vi "EnFlo_Tunnel_Display.vi"(4 "End Time":dbl, 5 "Start Time":dbl, 6 "Channel Values":dbl[](array[numeric]) format="%.3f", 7 "Ch names":string[](array[string])) -> ()   [LabVIEW 2021]
uses:
  Anemometry Sub Vis/Data_plotting_vis/File_Template_Clus.ctl
  Data plotting/subVIs/Dispose_Channel.ctl
  Anemometry Sub Vis/Controls/Global_mode.ctl
  Anemometry Sub Vis/Globals/Constants_global.vi
  Anemometry Sub Vis/Data_plotting_vis/Results_plotter_Global.vi
  <vilib>/gmath/NI_Gmath.lvlib
panel:
  out "Fan_Heater_2:Enable":bool
  out "Fan_Heater_1:Enable":bool
  out "EnFlo Lab:Heating Water:Temp":dbl format="%#.2g"
  out "Chiller_Pump Running":bool
  out "Inlet_Temp Average":dbl format="%#.2g"
  out "EnFlo_Tunnel:Power:Inlet_Door_Heaters":dbl format="%#.2g"
  out "Exit Heater Power %":dbl format="%#.2g"
  out "Averaging time (minutes)":dbl format="%#.1f"
  out "End time":timestamp format="%<%H:%M\n%x>T"
  out "Start time":timestamp format="%<%H:%M\n%x>T"
  out "Top Level":bool
  out "Loop number":i32
  out "Lateral profiles":cluster{"Y Axis Current":dbl[], dbl[]}[](graph)
  out "Setpoints":dbl[](array[numeric])
  in  "Subtract Setpoint?":bool
  out "Vert Disp (mm)  @ 14m":dbl
  out "Inlet St Dev":dbl format="%#.3g"
  out "Inlet mapping":dbl[][](graph)=[[0.00729, 0.18153463174730816, 0.17352738437348433, 1.6752433719500537, 8.231465735195274, 17.570357598383207, 23.099772817121426, 25.58386930448374, 25.31727725753219, 24.28926231541072, 18.717383219374323, 10.355253339797807, 2.7760273383248344, 0.3109897541921306, 0.08276881403435009, 0.06197], [0.04411, 0.1361526368018142, 0.04039202183336771, 1.5611636795339547, 8.176972694107874, 17.32000974741714, 24.257541358764026, 25.949153465972987, 26.01802540761648, 25.060373307424115, 18.284750328365213, 8.689831176707928, 2.642937641487066, 0.43219350072447926, -0.019957690739617468, 0.07351], [0.05478, 0.03446320268089581, 0.2086595806581808, 1.6919212249796047, 6.580368005180591, 14.333585185483123, 21.06810094963999, 23.709254571137723, 24.04768940379576, 21.01660820522005, 13.60443428327954, 6.2766496258038735, 1.7988963349022484, 0.2952877651784204, 0.05436788410934033, 0.1022], [0.04013, 0.06419557464541133, 0.2035068586120256, 1.3118741659450193, 4.7061387064566835, 9.009825946069038, 12.927700276268434, 17.003135081884164, 16.83885730812343, 12.902263313363814, 8.246161922417906, 4.035269404379355, 1.329605659745338, 0.24574055091433544, 0.012829784119986217, 0.08755], [0.04404, 0.022691144295571734, 0.19102098261858932, 0.8525411026079828, 2.2353542219792946, 3.966676465246214, 6.305347763088489, 8.17672908183636, 7.7348668140659, 5.703994479070454, 3.8329088824353237, 1.9256956625267279, 0.6611488869641811, 0.20508248283573002, 0.10119553469307395, 0.08441]]
  out "Floor Panels":cluster{"Array":dbl[], dbl[]}[](graph)
  in  "Averaging time (mins)":dbl=0.5 format="%.2f"
  in  "History in Minutes":dbl
  out "Strat":cluster{dbl[], dbl[]}[](graph)
  out "Des Air Temp":dbl format="%#.2g"
  out "Heat Extraction kW":dbl format="%#.2g"
  out "Lab Reference Temp":dbl format="%#.2g"
  out "Av Exit  Temp":dbl format="%#.2g"
  out "Exit Dem Temp":dbl format="%#.2g"
  out "Heat Exchanger Valve %":dbl format="%#.1f"
  out "Delta T":dbl format="%#.2g"
  out "Pump Speed %":dbl format="%#.0f"
  out "Meas Delta P":dbl format="%#.2g"
  out "Return Pressure":dbl format="%#.2g"
  out "Supply Pressure":dbl format="%#.2g"
  out "Max Motor Temp":dbl format="%#.1g"
  out "% Speed Tweak":dbl format="%#.2g"
  out "Shaft RPM":dbl format="%#.2g"
  out "Tunnel Speed  m/s":dbl format="%.3g"
  out "Uni Chilled water Temp":dbl format="%#.2g"
  out "Mixing Valve %":dbl format="%#.1f"
  out "Dem Temp":dbl
  out "Return Temp":dbl format="%#.2g"
  out "Supply Temp":dbl format="%#.2g"
  out "Floor_Cooling:Enable":bool
  out "Chiller_Pump:Enable":bool
  out "Panel Temps":cluster{"Array":dbl[], dbl[]}[](graph)
  in  "Stop Button":bool
  out "Heaters Enabled":bool
  out "Inlet Heaters":cluster{"yi":dbl[], dbl[]}[](graph)
  # "Chiller Pump Information"
  # "Chilled Water"
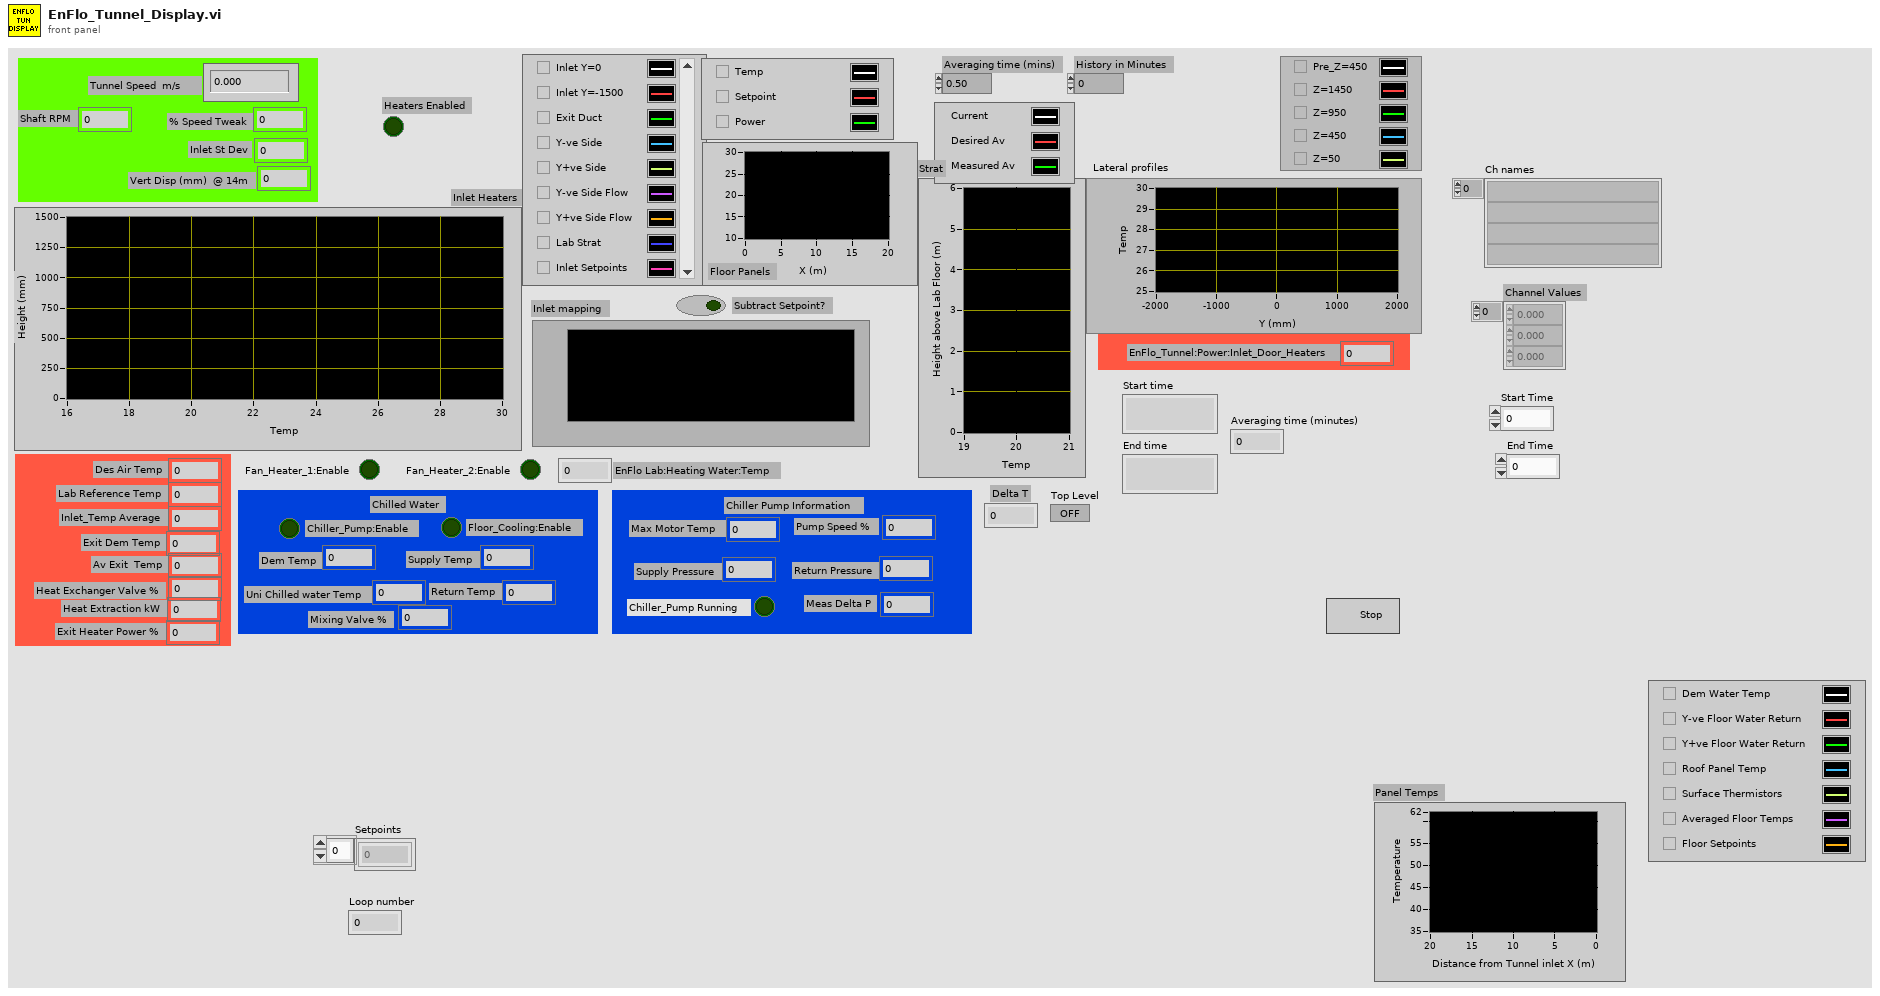
[diagram p1: front panel]
types:
  T1 = typedef "Global_mode.ctl" = enum16{"Read Global", "Load Global From File", "Write Global to File"}
  T2 = typedef "File_Template_Clus.ctl" = cluster{"Template Channel Name":string, "Description":string, "Tolerance":dbl, "Precision":string, "Folder level":string, "Source":string[], "Replace":string[], "Summarise":bool, "Min Value":string, "Maths":string, "Omit Rows Containing":string[], "Ignore When":string[], "Max Value":string, "Dispose":T3}
  T3 = typedef "Dispose_Channel.ctl" = enum16{"Always", "If Blank", "Never"}
  T4 = cluster{"X Max":dbl, "Y Max ":dbl, "X Scale":cluster{"Xo":dbl, "delta X":dbl}, "Y Scale":cluster{"Xo":dbl, "delta X":dbl}, "X Values":dbl[], "Y Values":dbl[], "Z Max":dbl, "Z Min":dbl}
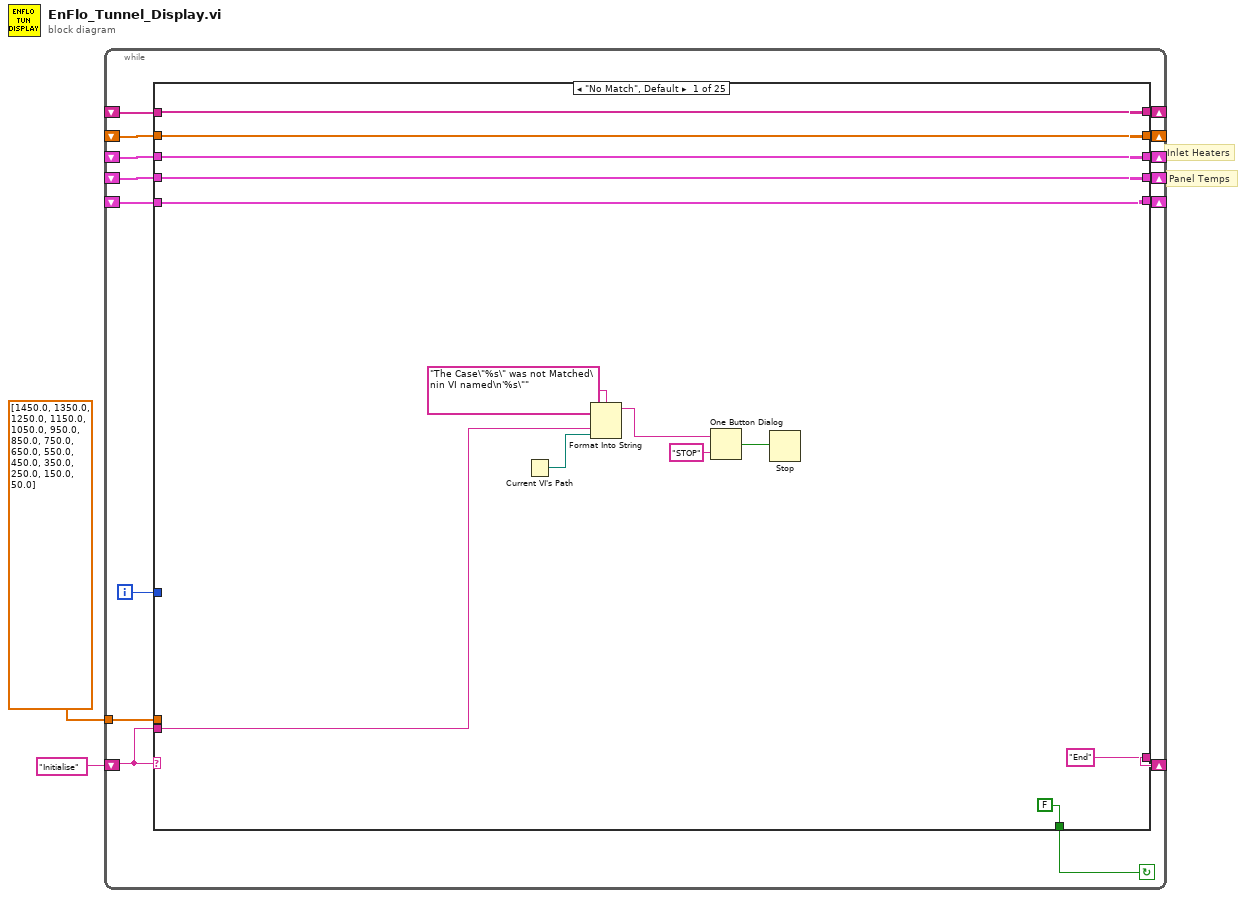
[diagram p0: block diagram]
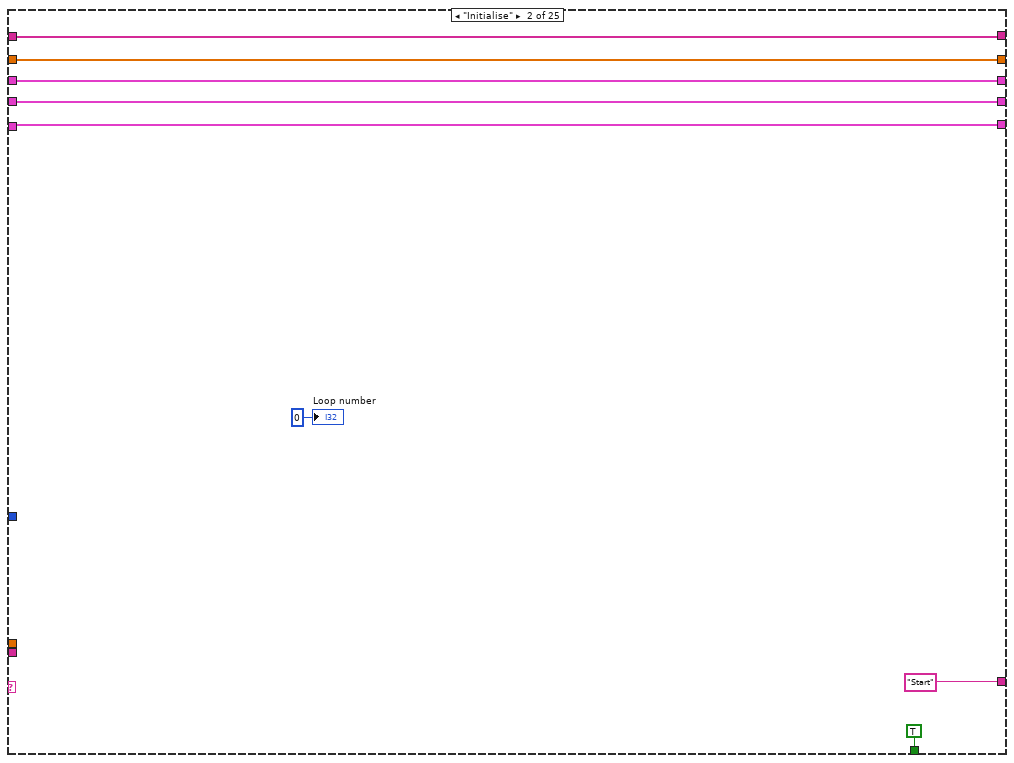
[diagram p2: hidden frame]
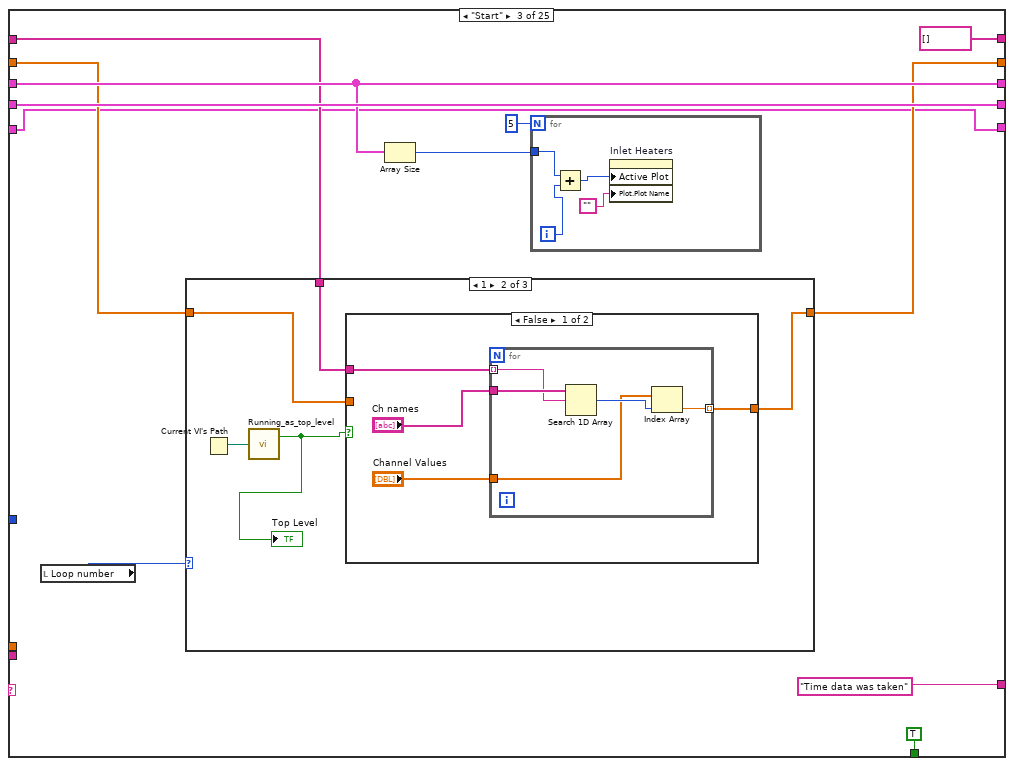
[diagram p3: hidden frame]
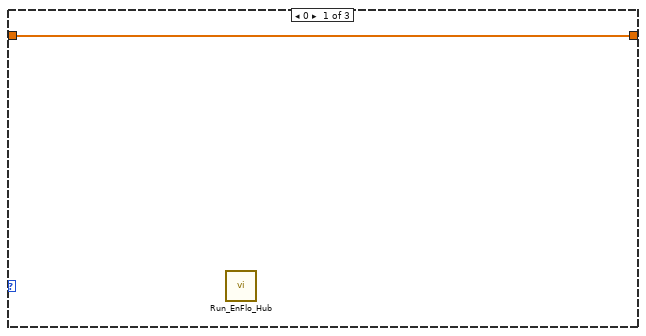
[diagram p4: hidden frame]
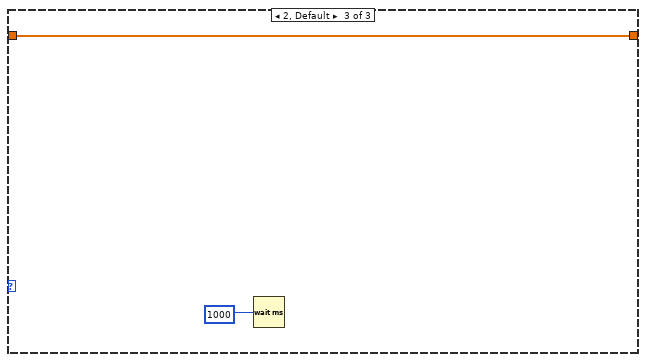
[diagram p6: hidden frame]
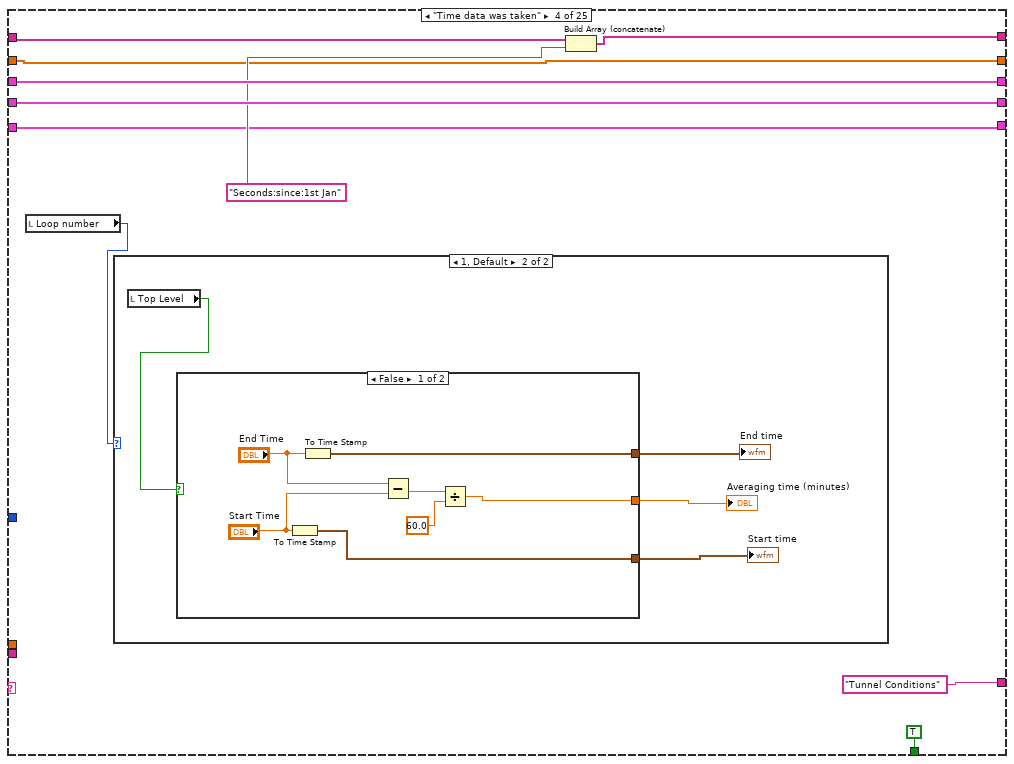
[diagram p7: hidden frame]
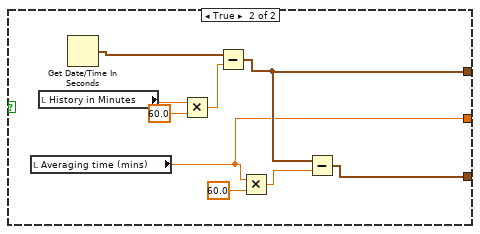
[diagram p9: hidden frame]
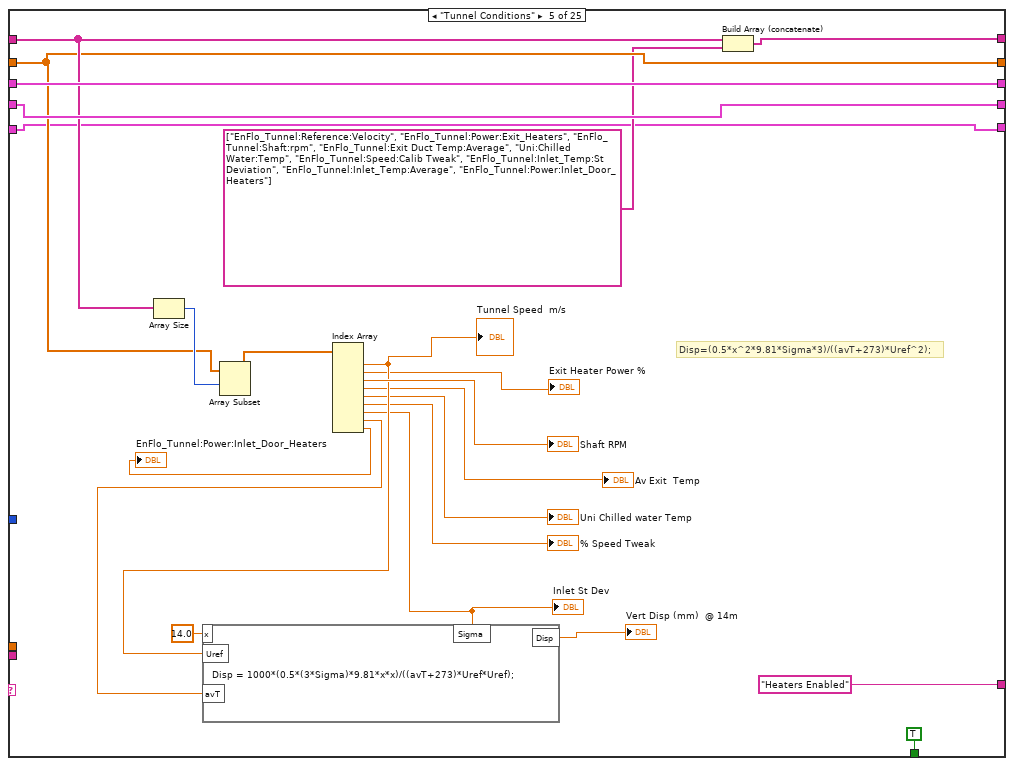
[diagram p10: hidden frame]
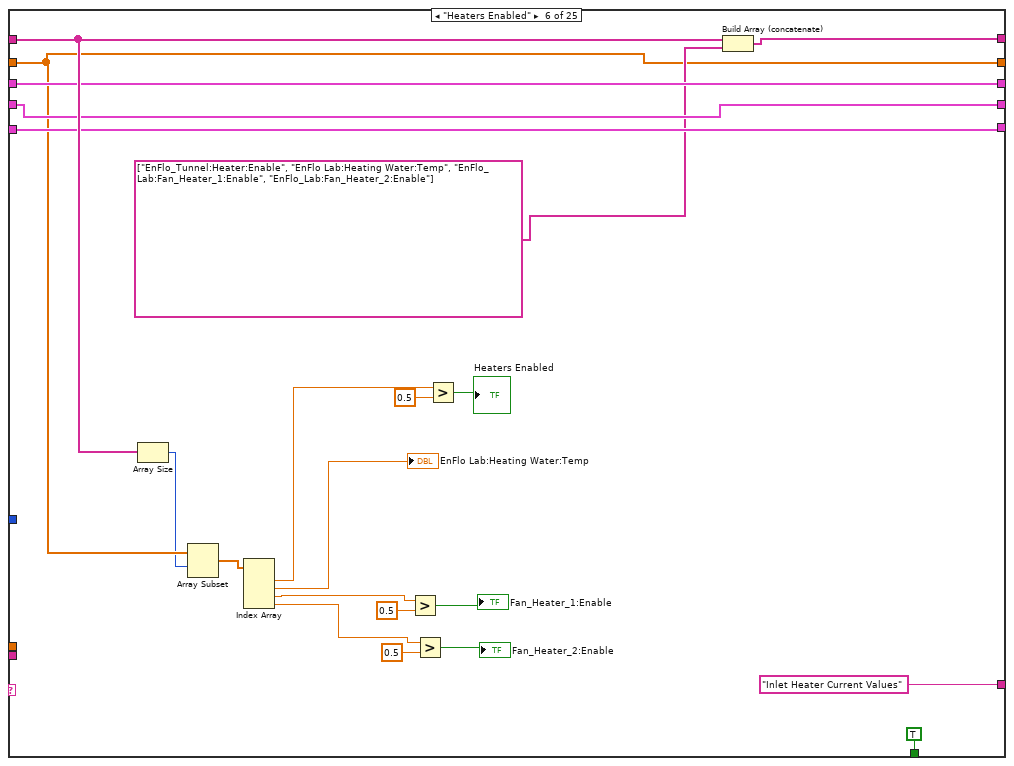
[diagram p11: hidden frame]
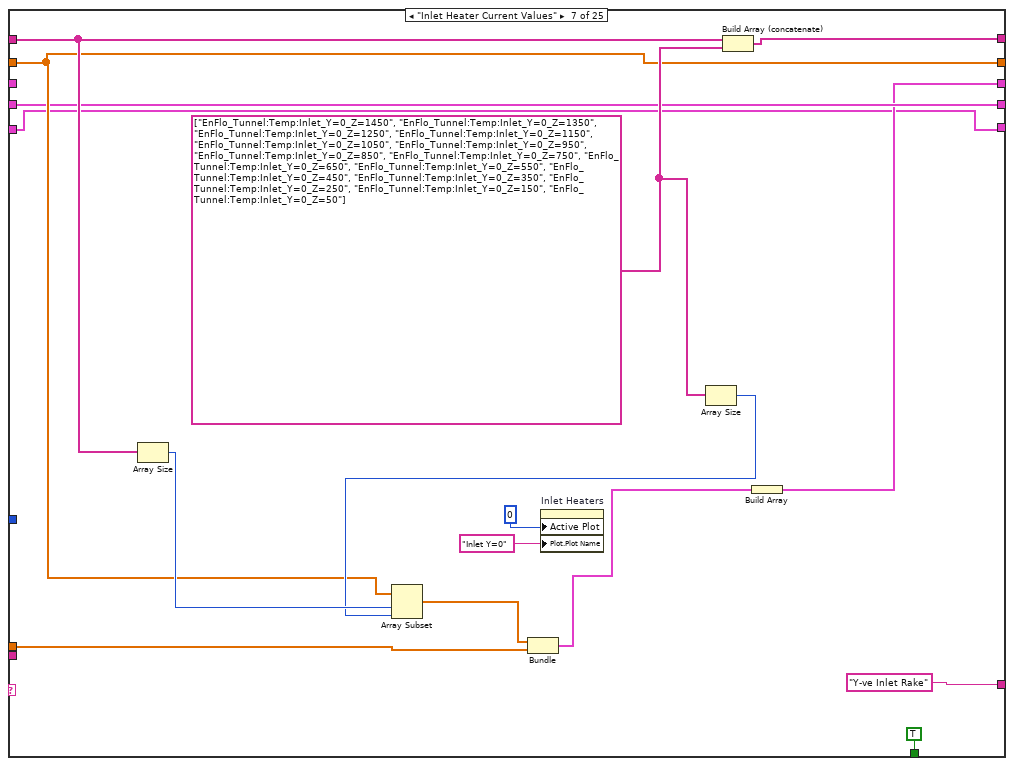
[diagram p12: hidden frame]
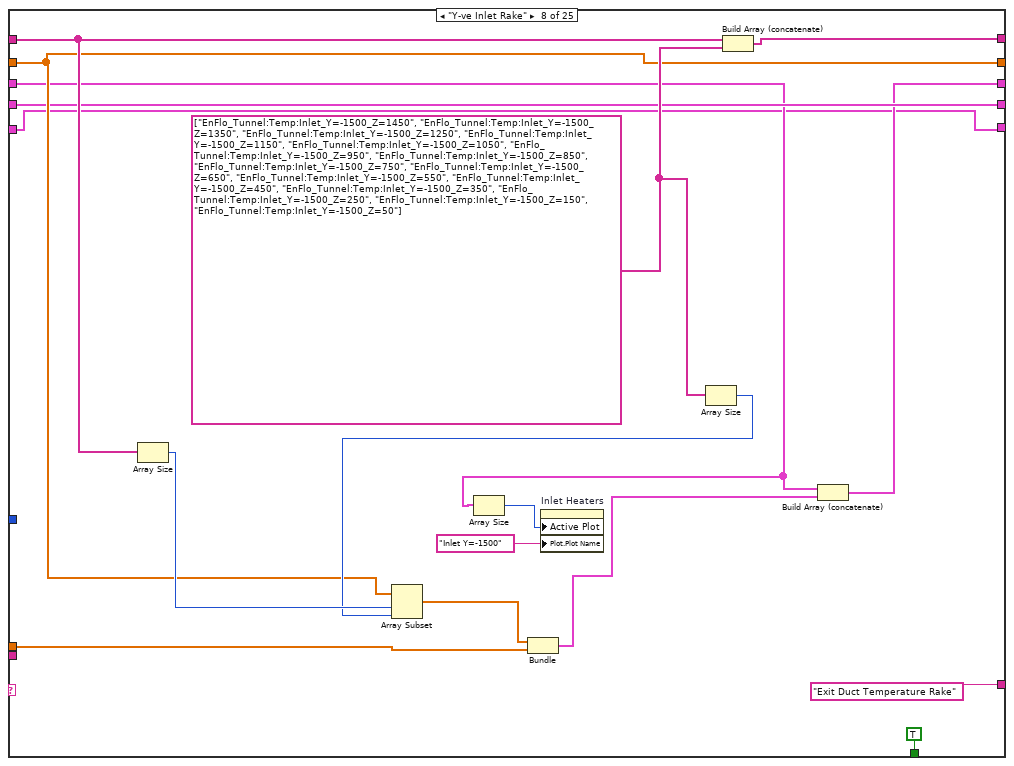
[diagram p13: hidden frame]
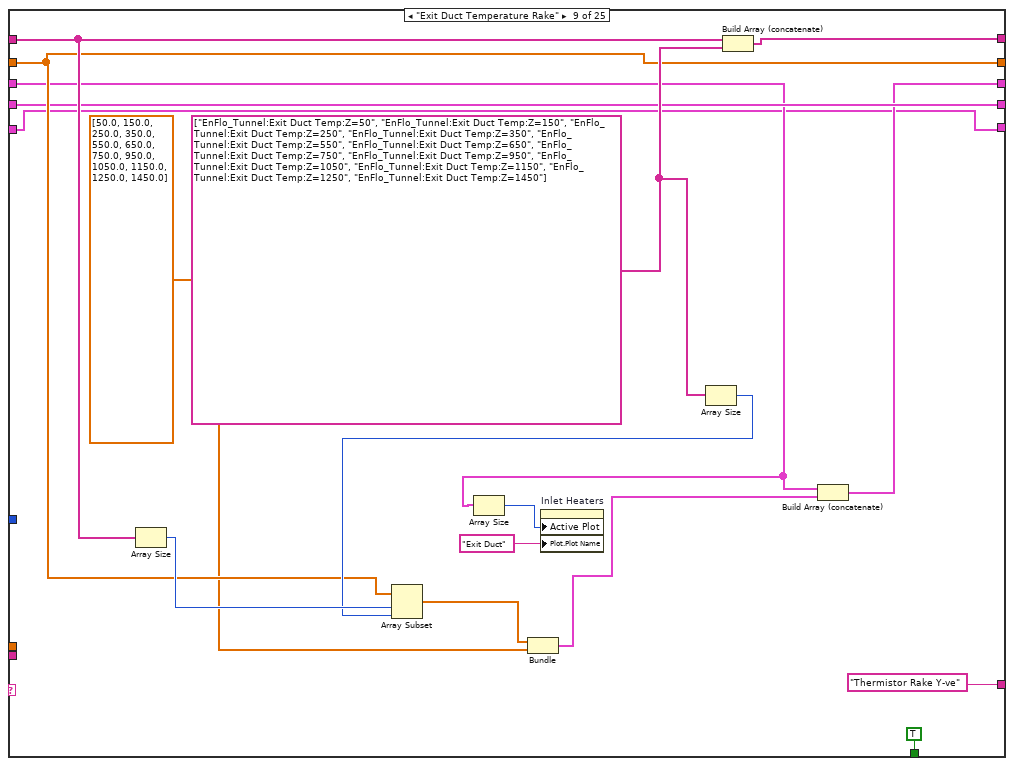
[diagram p14: hidden frame]
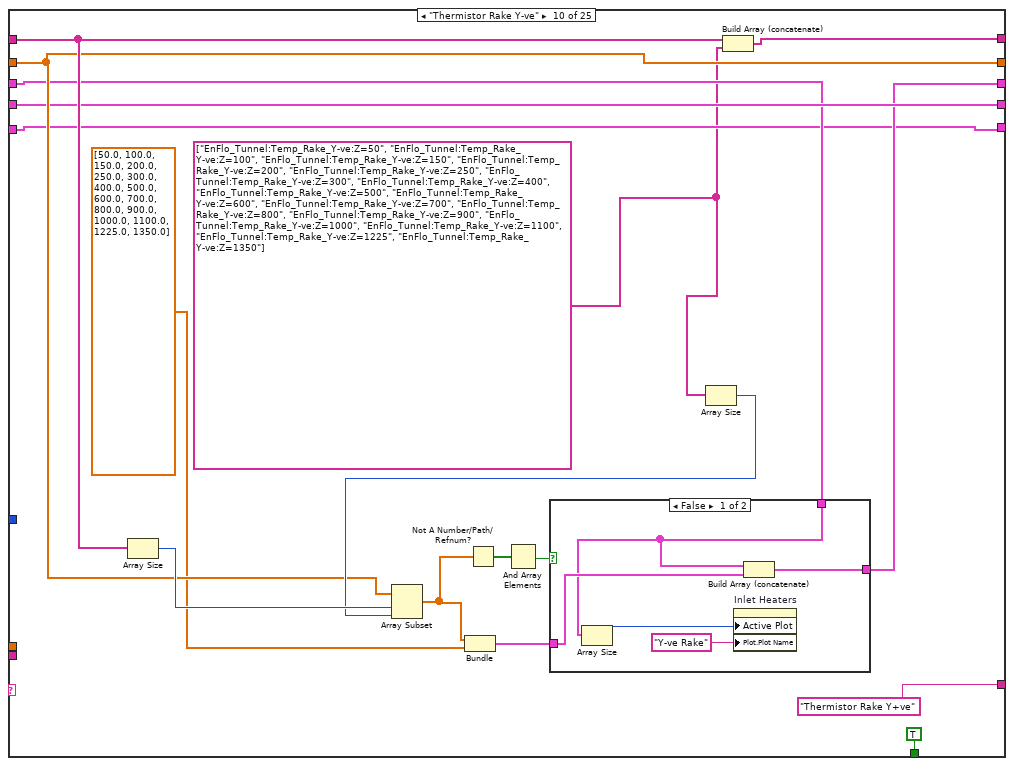
[diagram p15: hidden frame]
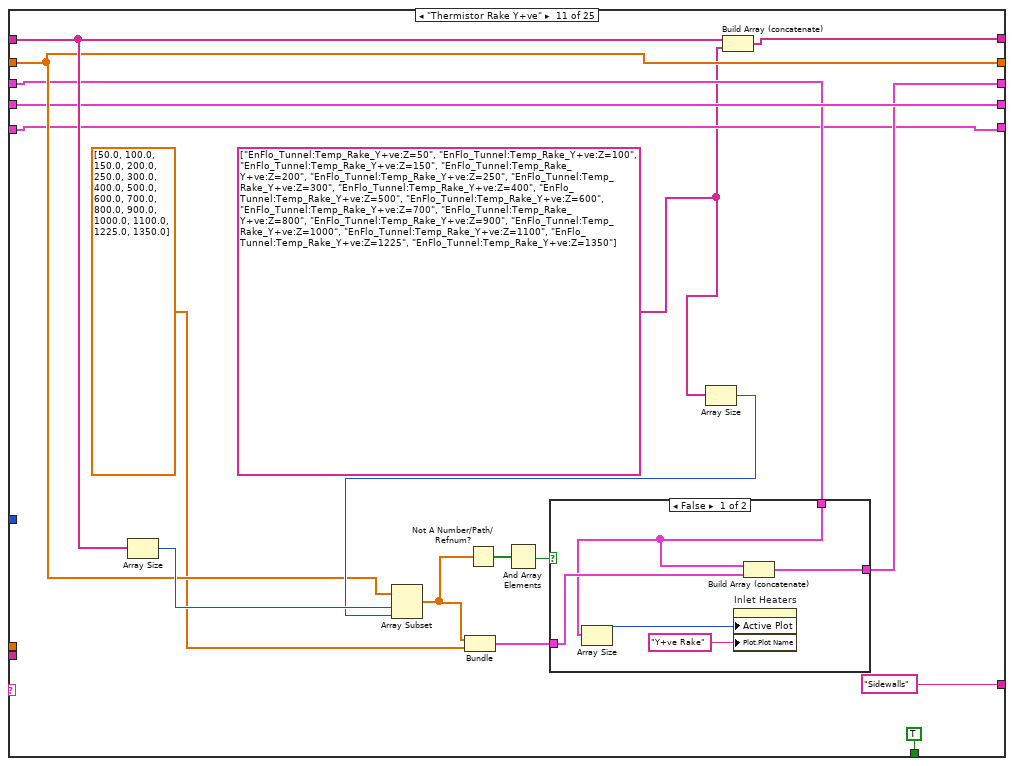
[diagram p17: hidden frame]
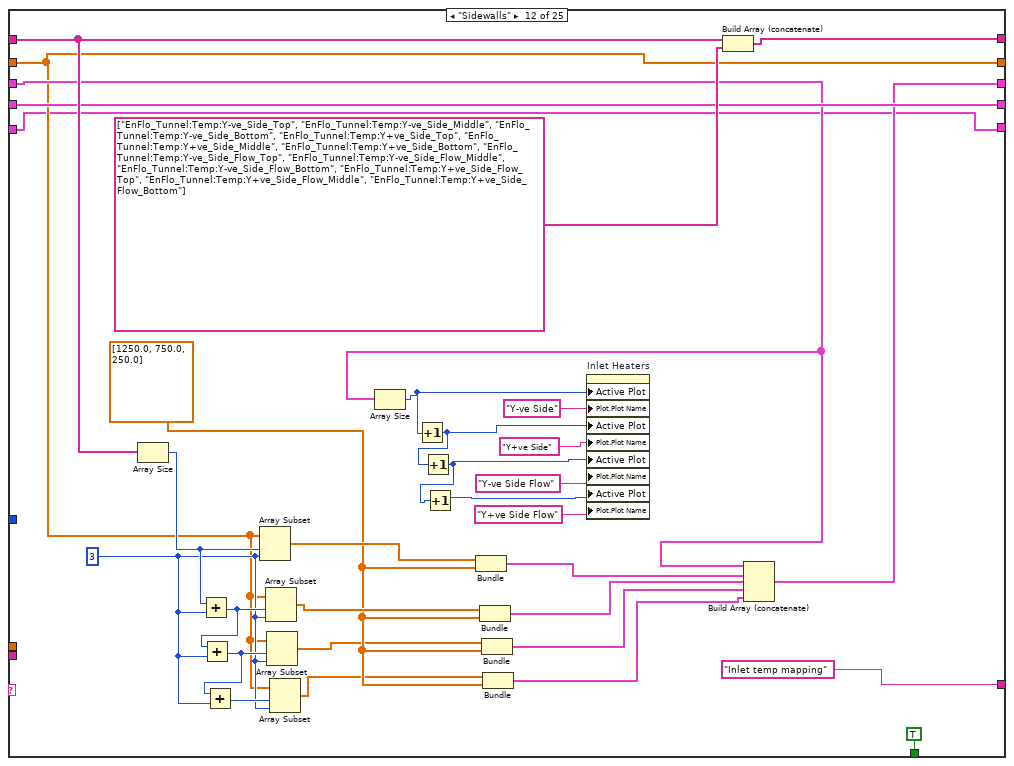
[diagram p19: hidden frame]
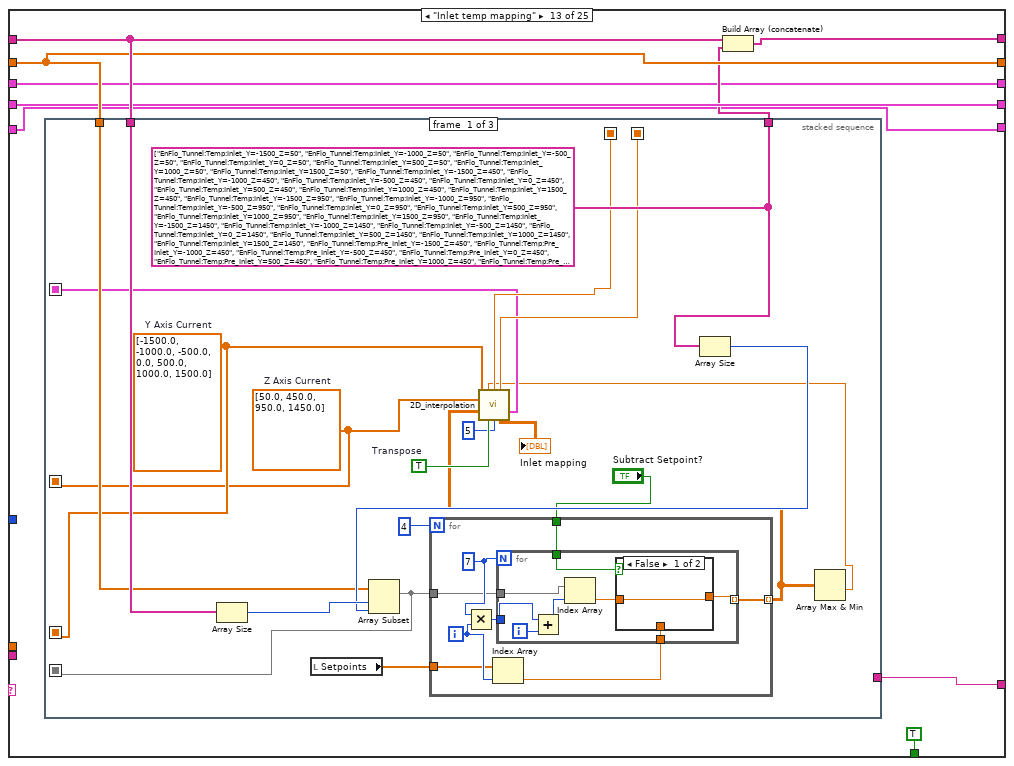
[diagram p20: hidden frame]
diagram:
  # "Panel Temps"
  # "Inlet Heaters"
  n1 = while {
    shift-right: [w15] -> _
    shift-left: "Initialise" -> [w16]
    shift-right: [w14] -> _
    shift-left: _ -> [w13]
    shift-right: [w11] -> _
    shift-left: _ -> [w12]
    shift-right: [w9] -> _
    shift-left: _ -> [w10]
    shift-right: [w8] -> _
    shift-left: _ -> [w7]
    tunnel: dbl[] [1450.0, 1350.0, 1250.0, 1150.0, 1050.0, 950.0, 850.0, 750.0, 650.0, 550.0, 450.0, 350.0, 250.0, 150.0, 50.0] -> [w5]
    shift-right: [w3] -> _
    shift-left: _ -> [w4]
    i -> [w6]
    stop <- w17 continue-if-true
    n2 = case shown="\"No Match\", Default" w16 {
      tunnel: [FALSE TRUE ("Top Level") TRUE TRUE ("Top Level") TRUE TRUE TRUE TRUE TRUE TRUE TRUE TRUE TRUE TRUE TRUE TRUE TRUE TRUE TRUE TRUE TRUE TRUE TRUE TRUE w606] -> w17
      tunnel: w16 -> [w24 _ _ _ _ _ _ _ _ _ _ _ _ _ _ _ _ _ _ _ _ _ _ _ _]
      tunnel: ["End" "Start" "Time data was taken" "Tunnel Conditions" "Heaters Enabled" "Inlet Heater Current Values" "Y-ve Inlet Rake" "Exit Duct Temperature Rake" "Thermistor Rake Y-ve" "Thermistor Rake Y+ve" "Sidewalls" "Inlet temp mapping" w275 "EnFlo_Tunnel Chilled Water info" "EnFlo_Tunnel:Floor_Cooling:Enable" "Floor Panels Return Temps" "Roof Panel Values" "Floor Panel Temps" "Floor Panel Setpoints" "Floor Panel Powers" "Lab Stratification" w513 "Inlet Heater Power Values" "Get Server Values" "Start"] -> w15
      tunnel: [w22 w34 string[] [] w79 w122 w143 w159 w176 w193 w211 w234 w271 w281 w362 w391 w404 w427 w457 w473 w490 w507 w546 w573 w593 w603] -> w14
      tunnel: w13 -> [w22 w34 w41 w78 w117 w142 w158 w175 w192 w210 w233 w270 w280 w361 w390 w403 w426 w456 w472 w489 w506 w545 w572 w592 w603]
      tunnel: w12 -> [w21 w35 w42 w75 w116 w134 w155 w172 w189 w207 w230 w245 w279 w358 w385 w400 w423 w453 w469 w486 w503 w532 w569 w589 _]
      tunnel: [w21 w35 w43 w75 w116 w134 w155 w172 w189 w207 w230 w245 w279 w358 w385 w400 w423 w453 w469 w486 w503 w532 w569 w589 w605] -> w11
      tunnel: w10 -> [w20 w38 w47 w82 w121 w141 _ w164 w182 w203 w226 w260 w276 w357 w389 w399 w421 w452 w468 w485 w502 w515 w560 w581 w601]
      tunnel: [w20 w38 w47 w82 w121 w141 w148 w167 w185 w204 w227 w266 w276 w357 w389 w399 w421 w452 w468 w485 w502 w536 w567 w585 w601] -> w9
      tunnel: w7 -> [w19 w37 w48 w81 w120 w137 w154 w171 w188 w206 w229 w269 w278 w353 w388 w395 _ w451 w464 w482 w499 w544 w566 w587 w602]
      tunnel: [w19 w37 w48 w81 w120 w137 w154 w171 w188 w206 w229 w269 w278 w353 w388 w395 w408 w450 w464 w482 w499 w544 w566 w587 w602] -> w8
      tunnel: w6 -> [_ _ _ _ _ _ _ _ _ _ _ _ _ _ _ _ _ _ _ _ _ _ _ _ _]
      tunnel: w5 -> [_ _ _ _ _ _ w152 w169 _ _ _ _ _ _ _ _ _ _ _ _ _ w518 w561 w586 _]
      tunnel: w4 -> [w18 w31 w39 w73 w110 w136 w146 w162 w180 w198 w221 w242 w274 w351 w368 w393 w406 w445 _ w479 w496 w511 w556 w578 w599]
      tunnel: [w18 w31 w39 w73 w110 w136 w146 w162 w180 w198 w221 w242 w274 w351 w368 w393 w406 w445 w462 w480 w497 w511 w556 w578 w599] -> w3
      frame "No Match", Default {
        n3 = Current VI's Path() -> (path=w29:path)
        n4 = Format Into String(format string="The Case\"%s\" was not Matched\nin VI named\n'%s\"" ("Format String"), w24, w29) -> (resulting string=w26:string)  [unwired: 2 in, 1 out]
        n5 = One Button Dialog(message=w26, button name ("OK")="STOP") -> (true=w28:bool)
        n6 = Stop(stop? (T)=w28) -> ()
      }
      frame "Initialise" {
        "Loop number" <- 0 ("Loop number")
      }
      frame "Start" {
        n7 = local read "Loop number"() -> (w44:i32)
        n8 = case shown="1" w44 {
          tunnel: [w55 w59 w71] -> w43
          tunnel: w42 -> [w55 w57 w71]
          tunnel: w41 -> [_ w60 _]
          frame 0 {
            n9 = call "Run_EnFlo_Hub.vi"() -> ()  [unwired: 7 in, 1 out]
          }
          frame 1 {
            n10 = Current VI's Path() -> (path=w58:path)
            n11 = call "Running_as_top_level.vi"("Vi path name"=w58) -> ("Top Level"=w56:bool)  [unwired: 1 out]
            "Top Level" <- w56
            n12 = case shown="False" w56 {
              tunnel: w60 -> [w63 _]
              tunnel: [w61 w70] -> w59
              tunnel: w57 -> [_ w70]
              frame False {
                n13 = for {
                  tunnel: "Ch names" -> [w69]
                  tunnel: w63 -> [w68] mode=indexing
                  tunnel: "Channel Values" -> [w66]
                  tunnel: [w65] -> w61 mode=indexing
                  n14 = Search 1D Array(1D array=w69, element=w68) -> (index of element=w67:i32)  [unwired: 1 in]
                  n15 = Index Array(array=w66, index=w67) -> (element=w65:dbl)
                }
              }
              frame True {
              }
            }
          }
          frame 2, Default {
            n16 = Wait (ms)(milliseconds to wait=u32 1000 ("millisecond timer value")) -> ()  [unwired: 1 out]
          }
        }
        n17 = Array Size(array=w47) -> (size(s)=w45:i32)
        n18 = for {
          N: 5 -> [_]
          tunnel: w45 -> [w54]
          i -> [w53]
          n19 = Add(x=w54, y=w53) -> (x+y=w52:i32)
          n20 = property on="Inlet Heaters" class="XYGraph (strict)"("Active Plot"=w52, "Plot.Plot Name"="") -> ()  [unwired: 2 in, 2 out]
        }
      }
      frame "Time data was taken" {
        n21 = local read "Loop number"() -> (w74:i32)
        n22 = case shown="1, Default" w74 {
          frame 0 {
          }
          frame 1, Default {
            n23 = local read "Top Level"() -> (w84:bool)
            n24 = case shown="False" w84 {
              tunnel: [w93 w100] -> w86
              tunnel: [w92 w101] -> w85
              tunnel: [w87 w94] -> w83
              frame False {
                n25 = To Time Stamp(1:"Start Time") -> (0:w93:timestamp)
                n26 = To Time Stamp(1:"End Time") -> (0:w92:timestamp)
                n27 = Subtract(x="End Time", y="Start Time") -> (x-y=w89:dbl)
                n28 = Divide(x=w89, y=60.0) -> (x/y=w87:dbl)
              }
              frame True {
                n29 = local read "Averaging time (mins)"() -> (w94:dbl)
                n30 = local read "History in Minutes"() -> (w99:dbl)
                n31 = Get Date/Time In Seconds() -> (seconds since 1Jan1904=w102:timestamp)
                n32 = Multiply(x=w99, y=60.0) -> (x*y=w97:dbl)
                n33 = Subtract(x=w102, y=w97) -> (x-y=w101:timestamp)
                n34 = Multiply(x=w94, y=60.0) -> (x*y=w95:dbl)
                n35 = Subtract(x=w101, y=w95) -> (x-y=w100:timestamp)
              }
            }
            "Start time" <- w86
            "End time" <- w85
            "Averaging time (minutes)" <- w83
          }
        }
        n36 = Build Array (concatenate)(w78, "Seconds:since:1st Jan") -> (w79:string[])
      }
      frame "Tunnel Conditions" {
        # "Disp=(0.5*x^2*9.81*Sigma*3)/((avT+273)*Uref^2);"
        n37 = Array Size(array=w117) -> (size(s)=w119:i32)
        n38 = Array Subset(array=w116, index=w119) -> (w118:dbl[])  [unwired: 1 in]
        n39 = Index Array(array=w118) -> (element #1=w112:dbl, element #2=→"Exit Heater Power %":dbl, element #3=→"Shaft RPM":dbl, element #4=→"Av Exit  Temp":dbl, element #5=→"Uni Chilled water Temp":dbl, element #6=→"% Speed Tweak":dbl, element #7=w105:dbl, element #8=w104:dbl, element #9=→"EnFlo_Tunnel:Power:Inlet_Door_Heaters":dbl)  [unwired: 9 in]
        "Tunnel Speed  m/s" <- w112
        "Inlet St Dev" <- w105
        n40 = formula code="Disp = 1000*(0.5*(3*Sigma)*9.81*x*x)/((avT+273)*Uref*Uref);"("x"=14.0 ("input variable"), "Uref"=w112, "Sigma"=w105, "avT"=w104) -> ("Disp"=→"Vert Disp (mm)  @ 14m":dbl)
        n41 = Build Array (concatenate)(w117, string[] ["EnFlo_Tunnel:Reference:Velocity", "EnFlo_Tunnel:Power:Exit_Heaters", "EnFlo_Tunnel:Shaft:rpm", "EnFlo_Tunnel:Exit Duct Temp:Average", "Uni:Chilled Water:Temp", "EnFlo_Tunnel:Speed:Calib Tweak", "EnFlo_Tunnel:Inlet_Temp:St Deviation", "EnFlo_Tunnel:Inlet_Temp:Average", "EnFlo_Tunnel:Power:Inlet_Door_Heaters"] ("subarray")) -> (w122:string[])
      }
      frame "Heaters Enabled" {
        n42 = Array Size(array=w142) -> (size(s)=w133:i32)
        n43 = Array Subset(array=w134, index=w133) -> (w132:dbl[])  [unwired: 1 in]
        n44 = Index Array(array=w132) -> (element #1=w140:dbl, element #2=→"EnFlo Lab:Heating Water:Temp":dbl, element #3=w128:dbl, element #4=w127:dbl)  [unwired: 4 in]
        n45 = Greater?(x=w128, y=0.5) -> (0:→"Fan_Heater_1:Enable":bool)
        n46 = Greater?(x=w127, y=0.5) -> (0:→"Fan_Heater_2:Enable":bool)
        n47 = Greater?(x=w140, y=0.5) -> (0:→"Heaters Enabled":bool)
        n48 = Build Array (concatenate)(w142, string[] ["EnFlo_Tunnel:Heater:Enable", "EnFlo Lab:Heating Water:Temp", "EnFlo_Lab:Fan_Heater_1:Enable", "EnFlo_Lab:Fan_Heater_2:Enable"]) -> (w143:string[])
      }
      frame "Inlet Heater Current Values" {
        w160 = string[] ["EnFlo_Tunnel:Temp:Inlet_Y=0_Z=1450", "EnFlo_Tunnel:Temp:Inlet_Y=0_Z=1350", "EnFlo_Tunnel:Temp:Inlet_Y=0_Z=1250", "EnFlo_Tunnel:Temp:Inlet_Y=0_Z=1150", "EnFlo_Tunnel:Temp:Inlet_Y=0_Z=1050", "EnFlo_Tunnel:Temp:Inlet_Y=0_Z=950", "EnFlo_Tunnel:Temp:Inlet_Y=0_Z=850", "EnFlo_Tunnel:Temp:Inlet_Y=0_Z=750", "EnFlo_Tunnel:Temp:Inlet_Y=0_Z=650", "EnFlo_Tunnel:Temp:Inlet_Y=0_Z=550", "EnFlo_Tunnel:Temp:Inlet_Y=0_Z=450", "EnFlo_Tunnel:Temp:Inlet_Y=0_Z=350", "EnFlo_Tunnel:Temp:Inlet_Y=0_Z=250", "EnFlo_Tunnel:Temp:Inlet_Y=0_Z=150", "EnFlo_Tunnel:Temp:Inlet_Y=0_Z=50"] ("subarray")
        n49 = Array Size(array=w158) -> (size(s)=w157:i32)
        n50 = property on="Inlet Heaters" class="XYGraph (strict)"("Active Plot"=u32 0, "Plot.Plot Name"="Inlet Y=0") -> ()  [unwired: 2 in, 2 out]
        n51 = Array Size(array=w160) -> (size(s)=w156:i32)
        n52 = Array Subset(array=w155, index=w157, length=w156) -> (w153:dbl[])
        n53 = Bundle(w153, w152) -> (w149:cluster{dbl[], dbl[]})  [unwired: 1 in]
        n54 = Build Array (concatenate)(w158, w160) -> (w159:string[])
        n55 = Build Array(w149) -> (w148:cluster{dbl[], dbl[]}[])
      }
      frame "Y-ve Inlet Rake" {
        w177 = string[] ["EnFlo_Tunnel:Temp:Inlet_Y=-1500_Z=1450", "EnFlo_Tunnel:Temp:Inlet_Y=-1500_Z=1350", "EnFlo_Tunnel:Temp:Inlet_Y=-1500_Z=1250", "EnFlo_Tunnel:Temp:Inlet_Y=-1500_Z=1150", "EnFlo_Tunnel:Temp:Inlet_Y=-1500_Z=1050", "EnFlo_Tunnel:Temp:Inlet_Y=-1500_Z=950", "EnFlo_Tunnel:Temp:Inlet_Y=-1500_Z=850", "EnFlo_Tunnel:Temp:Inlet_Y=-1500_Z=750", "EnFlo_Tunnel:Temp:Inlet_Y=-1500_Z=650", "EnFlo_Tunnel:Temp:Inlet_Y=-1500_Z=550", "EnFlo_Tunnel:Temp:Inlet_Y=-1500_Z=450", "EnFlo_Tunnel:Temp:Inlet_Y=-1500_Z=350", "EnFlo_Tunnel:Temp:Inlet_Y=-1500_Z=250", "EnFlo_Tunnel:Temp:Inlet_Y=-1500_Z=150", "EnFlo_Tunnel:Temp:Inlet_Y=-1500_Z=50"] ("subarray")
        n56 = Array Size(array=w175) -> (size(s)=w174:i32)
        n57 = Array Size(array=w164) -> (size(s)=w163:i32)
        n58 = property on="Inlet Heaters" class="XYGraph (strict)"("Active Plot"=w163, "Plot.Plot Name"="Inlet Y=-1500") -> ()  [unwired: 2 in, 2 out]
        n59 = Array Size(array=w177) -> (size(s)=w173:i32)
        n60 = Array Subset(array=w172, index=w174, length=w173) -> (w170:dbl[])
        n61 = Bundle(w170, w169) -> (w165:cluster{dbl[], dbl[]})  [unwired: 1 in]
        n62 = Build Array (concatenate)(w175, w177) -> (w176:string[])
        n63 = Build Array (concatenate)(w164, w165) -> (w167:cluster{"yi":dbl[], dbl[]}[])
      }
      frame "Exit Duct Temperature Rake" {
        w194 = string[] ["EnFlo_Tunnel:Exit Duct Temp:Z=50", "EnFlo_Tunnel:Exit Duct Temp:Z=150", "EnFlo_Tunnel:Exit Duct Temp:Z=250", "EnFlo_Tunnel:Exit Duct Temp:Z=350", "EnFlo_Tunnel:Exit Duct Temp:Z=550", "EnFlo_Tunnel:Exit Duct Temp:Z=650", "EnFlo_Tunnel:Exit Duct Temp:Z=750", "EnFlo_Tunnel:Exit Duct Temp:Z=950", "EnFlo_Tunnel:Exit Duct Temp:Z=1050", "EnFlo_Tunnel:Exit Duct Temp:Z=1150", "EnFlo_Tunnel:Exit Duct Temp:Z=1250", "EnFlo_Tunnel:Exit Duct Temp:Z=1450"] ("subarray")
        n64 = Array Size(array=w192) -> (size(s)=w191:i32)
        n65 = Array Size(array=w182) -> (size(s)=w181:i32)
        n66 = property on="Inlet Heaters" class="XYGraph (strict)"("Active Plot"=w181, "Plot.Plot Name"="Exit Duct") -> ()  [unwired: 2 in, 2 out]
        n67 = Array Size(array=w194) -> (size(s)=w190:i32)
        n68 = Array Subset(array=w189, index=w191, length=w190) -> (w187:dbl[])
        n69 = Bundle(w187, dbl[] [50.0, 150.0, 250.0, 350.0, 550.0, 650.0, 750.0, 950.0, 1050.0, 1150.0, 1250.0, 1450.0]) -> (w183:cluster{dbl[], dbl[]})  [unwired: 1 in]
        n70 = Build Array (concatenate)(w192, w194) -> (w193:string[])
        n71 = Build Array (concatenate)(w182, w183) -> (w185:cluster{"yi":dbl[], dbl[]}[])
      }
      frame "Thermistor Rake Y-ve" {
        w197 = string[] ["EnFlo_Tunnel:Temp_Rake_Y-ve:Z=50", "EnFlo_Tunnel:Temp_Rake_Y-ve:Z=100", "EnFlo_Tunnel:Temp_Rake_Y-ve:Z=150", "EnFlo_Tunnel:Temp_Rake_Y-ve:Z=200", "EnFlo_Tunnel:Temp_Rake_Y-ve:Z=250", "EnFlo_Tunnel:Temp_Rake_Y-ve:Z=300", "EnFlo_Tunnel:Temp_Rake_Y-ve:Z=400", "EnFlo_Tunnel:Temp_Rake_Y-ve:Z=500", "EnFlo_Tunnel:Temp_Rake_Y-ve:Z=600", "EnFlo_Tunnel:Temp_Rake_Y-ve:Z=700", "EnFlo_Tunnel:Temp_Rake_Y-ve:Z=800", "EnFlo_Tunnel:Temp_Rake_Y-ve:Z=900", "EnFlo_Tunnel:Temp_Rake_Y-ve:Z=1000", "EnFlo_Tunnel:Temp_Rake_Y-ve:Z=1100", "EnFlo_Tunnel:Temp_Rake_Y-ve:Z=1225", "EnFlo_Tunnel:Temp_Rake_Y-ve:Z=1350"] ("Sub set")
        n72 = Array Size(array=w210) -> (size(s)=w209:i32)
        n73 = Array Size(array=w197) -> (size(s)=w208:i32)
        n74 = Array Subset(array=w207, index=w209, length=w208) -> (w202:dbl[])
        n75 = Bundle(w202, dbl[] [50.0, 100.0, 150.0, 200.0, 250.0, 300.0, 400.0, 500.0, 600.0, 700.0, 800.0, 900.0, 1000.0, 1100.0, 1225.0, 1350.0]) -> (w199:cluster{dbl[], dbl[]})  [unwired: 1 in]
        n76 = Not A Number/Path/Refnum?(number/path/refnum=w202) -> (NaN/Path/Refnum?=w201:bool[])
        n77 = And Array Elements(Boolean array=w201) -> (logical AND=w200:bool)
        n78 = case shown="False" w200 {
          tunnel: [w217 w218] -> w204
          tunnel: w203 -> [w213 w218]
          tunnel: w199 -> [w216 _]
          frame False {
            n79 = Array Size(array=w213) -> (size(s)=w214:i32)
            n80 = property on="Inlet Heaters" class="XYGraph (strict)"("Active Plot"=w214, "Plot.Plot Name"="Y-ve Rake") -> ()  [unwired: 2 in, 2 out]
            n81 = Build Array (concatenate)(w213, w216) -> (w217:cluster{"yi":dbl[], dbl[]}[])
          }
          frame True {
          }
        }
        n82 = Build Array (concatenate)(w210, w197) -> (w211:string[])
      }
      frame "Thermistor Rake Y+ve" {
        w219 = string[] ["EnFlo_Tunnel:Temp_Rake_Y+ve:Z=50", "EnFlo_Tunnel:Temp_Rake_Y+ve:Z=100", "EnFlo_Tunnel:Temp_Rake_Y+ve:Z=150", "EnFlo_Tunnel:Temp_Rake_Y+ve:Z=200", "EnFlo_Tunnel:Temp_Rake_Y+ve:Z=250", "EnFlo_Tunnel:Temp_Rake_Y+ve:Z=300", "EnFlo_Tunnel:Temp_Rake_Y+ve:Z=400", "EnFlo_Tunnel:Temp_Rake_Y+ve:Z=500", "EnFlo_Tunnel:Temp_Rake_Y+ve:Z=600", "EnFlo_Tunnel:Temp_Rake_Y+ve:Z=700", "EnFlo_Tunnel:Temp_Rake_Y+ve:Z=800", "EnFlo_Tunnel:Temp_Rake_Y+ve:Z=900", "EnFlo_Tunnel:Temp_Rake_Y+ve:Z=1000", "EnFlo_Tunnel:Temp_Rake_Y+ve:Z=1100", "EnFlo_Tunnel:Temp_Rake_Y+ve:Z=1225", "EnFlo_Tunnel:Temp_Rake_Y+ve:Z=1350"] ("Sub set")
        n83 = Array Size(array=w233) -> (size(s)=w232:i32)
        n84 = Array Size(array=w219) -> (size(s)=w231:i32)
        n85 = Array Subset(array=w230, index=w232, length=w231) -> (w225:dbl[])
        n86 = Bundle(w225, dbl[] [50.0, 100.0, 150.0, 200.0, 250.0, 300.0, 400.0, 500.0, 600.0, 700.0, 800.0, 900.0, 1000.0, 1100.0, 1225.0, 1350.0]) -> (w222:cluster{dbl[], dbl[]})  [unwired: 1 in]
        n87 = Not A Number/Path/Refnum?(number/path/refnum=w225) -> (NaN/Path/Refnum?=w224:bool[])
        n88 = And Array Elements(Boolean array=w224) -> (logical AND=w223:bool)
        n89 = case shown="False" w223 {
          tunnel: [w240 w241] -> w227
          tunnel: w226 -> [w236 w241]
          tunnel: w222 -> [w239 _]
          frame False {
            n90 = Array Size(array=w236) -> (size(s)=w237:i32)
            n91 = property on="Inlet Heaters" class="XYGraph (strict)"("Active Plot"=w237, "Plot.Plot Name"="Y+ve Rake") -> ()  [unwired: 2 in, 2 out]
            n92 = Build Array (concatenate)(w236, w239) -> (w240:cluster{"yi":dbl[], dbl[]}[])
          }
          frame True {
          }
        }
        n93 = Build Array (concatenate)(w233, w219) -> (w234:string[])
      }
      frame "Sidewalls" {
        w248 = dbl[] [1250.0, 750.0, 250.0]
        w249 = 3 ("length")
        n94 = Array Size(array=w270) -> (size(s)=w265:i32)
        n95 = Add(x=w265, y=w249) -> (x+y=w251:i32)
        n96 = Add(x=w251, y=w249) -> (x+y=w250:i32)
        n97 = Add(x=w250, y=w249) -> (x+y=w252:i32)
        n98 = Array Subset(array=w245, index=w265, length=w249) -> (w264:dbl[])
        n99 = Array Subset(array=w245, index=w251, length=w249) -> (w263:dbl[])
        n100 = Array Subset(array=w245, index=w250, length=w249) -> (w247:dbl[])
        n101 = Array Subset(array=w245, index=w252, length=w249) -> (w246:dbl[])
        n102 = Array Size(array=w260) -> (size(s)=w258:i32)
        n103 = Increment(x=w258) -> (x+1=w255:i32)
        n104 = Increment(x=w255) -> (x+1=w253:i32)
        n105 = Increment(x=w253) -> (x+1=w254:i32)
        n106 = Bundle(w264, w248) -> (w267:cluster{dbl[], dbl[]})  [unwired: 1 in]
        n107 = Bundle(w263, w248) -> (w262:cluster{dbl[], dbl[]})  [unwired: 1 in]
        n108 = Bundle(w247, w248) -> (w244:cluster{dbl[], dbl[]})  [unwired: 1 in]
        n109 = Bundle(w246, w248) -> (w243:cluster{dbl[], dbl[]})  [unwired: 1 in]
        n110 = property on="Inlet Heaters" class="XYGraph (strict)"("Active Plot"=w258, "Plot.Plot Name"="Y-ve Side", "Active Plot"=w255, "Plot.Plot Name"="Y+ve Side", "Active Plot"=w253, "Plot.Plot Name"="Y-ve Side Flow", "Active Plot"=w254, "Plot.Plot Name"="Y+ve Side Flow") -> ()  [unwired: 2 in, 2 out]
        n111 = Build Array (concatenate)(w270, string[] ["EnFlo_Tunnel:Temp:Y-ve_Side_Top", "EnFlo_Tunnel:Temp:Y-ve_Side_Middle", "EnFlo_Tunnel:Temp:Y-ve_Side_Bottom", "EnFlo_Tunnel:Temp:Y+ve_Side_Top", "EnFlo_Tunnel:Temp:Y+ve_Side_Middle", "EnFlo_Tunnel:Temp:Y+ve_Side_Bottom", "EnFlo_Tunnel:Temp:Y-ve_Side_Flow_Top", "EnFlo_Tunnel:Temp:Y-ve_Side_Flow_Middle", "EnFlo_Tunnel:Temp:Y-ve_Side_Flow_Bottom", "EnFlo_Tunnel:Temp:Y+ve_Side_Flow_Top", "EnFlo_Tunnel:Temp:Y+ve_Side_Flow_Middle", "EnFlo_Tunnel:Temp:Y+ve_Side_Flow_Bottom"] ("subarray")) -> (w271:string[])
        n112 = Build Array (concatenate)(w260, w267, w262, w244, w243) -> (w266:cluster{"yi":dbl[], dbl[]}[])
      }
      frame "Inlet temp mapping" {
        n113 = stacked-sequence {
          seq-local: [w293 _ _] -> [_ w330 _]
          seq-local: [w292 _ _] -> [_ w331 _]
          seq-local: [w291 _ _] -> [_ w326 _]
          seq-local: [w285 _ _] -> [_ _ w341]
          seq-local: [w284 _ _] -> [_ _ w342]
          seq-local: [w283 _ _] -> [_ _ _]
          tunnel: w280 -> [w301 _ _]
          tunnel: w279 -> [w298 _ _]
          tunnel: [w297 _ _] -> w277
          tunnel: [_ "EnFlo_Tunnel:Chiller_Pump:Enable" _] -> w275
          frame #0 {
            w295 = TRUE  # Transpose
            w283 = dbl[] [50.0, 450.0, 950.0, 1450.0]  # Z Axis Current
            w284 = dbl[] [-1500.0, -1000.0, -500.0, 0.0, 500.0, 1000.0, 1500.0]  # Y Axis Current
            w297 = string[] ["EnFlo_Tunnel:Temp:Inlet_Y=-1500_Z=50", "EnFlo_Tunnel:Temp:Inlet_Y=-1000_Z=50", "EnFlo_Tunnel:Temp:Inlet_Y=-500_Z=50", "EnFlo_Tunnel:Temp:Inlet_Y=0_Z=50", "EnFlo_Tunnel:Temp:Inlet_Y=500_Z=50", "EnFlo_Tunnel:Temp:Inlet_Y=1000_Z=50", "EnFlo_Tunnel:Temp:Inlet_Y=1500_Z=50", "EnFlo_Tunnel:Temp:Inlet_Y=-1500_Z=450", "EnFlo_Tunnel:Temp:Inlet_Y=-1000_Z=450", "EnFlo_Tunnel:Temp:Inlet_Y=-500_Z=450", "EnFlo_Tunnel:Temp:Inlet_Y=0_Z=450", "EnFlo_Tunnel:Temp:Inlet_Y=500_Z=450", "EnFlo_Tunnel:Temp:Inlet_Y=1000_Z=450", "EnFlo_Tunnel:Temp:Inlet_Y=1500_Z=450", "EnFlo_Tunnel:Temp:Inlet_Y=-1500_Z=950", "EnFlo_Tunnel:Temp:Inlet_Y=-1000_Z=950", "EnFlo_Tunnel:Temp:Inlet_Y=-500_Z=950", "EnFlo_Tunnel:Temp:Inlet_Y=0_Z=950", "EnFlo_Tunnel:Temp:Inlet_Y=500_Z=950", "EnFlo_Tunnel:Temp:Inlet_Y=1000_Z=950", "EnFlo_Tunnel:Temp:Inlet_Y=1500_Z=950", "EnFlo_Tunnel:Temp:Inlet_Y=-1500_Z=1450", "EnFlo_Tunnel:Temp:Inlet_Y=-1000_Z=1450", "EnFlo_Tunnel:Temp:Inlet_Y=-500_Z=1450", "EnFlo_Tunnel:Temp:Inlet_Y=0_Z=1450", "EnFlo_Tunnel:Temp:Inlet_Y=500_Z=1450", "EnFlo_Tunnel:Temp:Inlet_Y=1000_Z=1450", "EnFlo_Tunnel:Temp:Inlet_Y=1500_Z=1450", "EnFlo_Tunnel:Temp:Pre_Inlet_Y=-1500_Z=450", "EnFlo_Tunnel:Temp:Pre_Inlet_Y=-1000_Z=450", "EnFlo_Tunnel:Temp:Pre_Inlet_Y=-500_Z=450", "EnFlo_Tunnel:Temp:Pre_Inlet_Y=0_Z=450", "EnFlo_Tunnel:Temp:Pre_Inlet_Y=500_Z=450", "EnFlo_Tunnel:Temp:Pre_Inlet_Y=1000_Z=450", "EnFlo_Tunnel:Temp:Pre_Inlet_Y=1500_Z=450"] ("subarray")
            n114 = Array Size(array=w301) -> (size(s)=w300:i32)
            n115 = local read "Setpoints"() -> (w289:dbl[])
            n116 = Array Size(array=w297) -> (size(s)=w299:i32)
            n117 = Array Subset(array=w298, index=w300, length=w299) -> (w285:dbl[])
            n118 = for {
              N: 4 -> [_]
              tunnel: [w307] -> w287 mode=indexing
              tunnel: w289 -> [w305]
              tunnel: "Subtract Setpoint?" -> [w304]
              tunnel: w285 -> [w302]
              i -> [w306]
              w309 = 7
              n119 = Multiply(x=w309, y=w306) -> (x*y=w308:i32)
              n120 = Index Array(array=w305, index=w306) -> (element=w303:dbl)
              n121 = for {
                N: w309 -> [_]
                tunnel: w308 -> [w316]
                tunnel: w302 -> [w314]
                tunnel: [w310] -> w307 mode=indexing
                tunnel: w304 -> [w313]
                tunnel: w303 -> [w311]
                i -> [w317]
                n122 = Add(x=w316, y=w317) -> (x+y=w315:i32)
                n123 = Index Array(array=w314, index=w315) -> (element=w312:dbl)
                n124 = case shown="False" w313 {
                  tunnel: w312 -> [w318 w321]
                  tunnel: w311 -> [_ w320]
                  tunnel: [w318 w319] -> w310
                  frame False {
                  }
                  frame True {
                    n125 = Subtract(x=w321, y=w320) -> (x-y=w319:dbl)
                  }
                }
              }
            }
            n126 = Array Max & Min(array=w287) -> (min value=w286:dbl)  [unwired: 3 out]
            n127 = call "2D_interpolation.vi"("X Axis Current"=w284, "Min Z Value In"=w286, "Y axis Current"=w283, "Plot In"=w287, "Transpose"=w295, "Point Size"=5) -> ("min Z value"=w293:dbl, "max Z value"=w292:dbl, "Axis info"=w291:T4, "Plot Out"=→"Inlet mapping":dbl[][])  [unwired: 2 in, 4 out]
          }
          frame #1 {
            w327 = u8 0 ("X Scale.Display Format:Precision")
            n128 = Bundle("max Z value"=w331, u32 16721152) -> (w334:cluster{"max Z value":dbl, u32})  [unwired: 1 out]
            n129 = Bundle("min Z value"=w330, u32 3743) -> (w335:cluster{"min Z value":dbl, u32})  [unwired: 1 out]
            n130 = Unbundle By Name(w326) -> ("Y Scale"=w325:cluster{"Xo":dbl, "delta X":dbl}, "Y Max"=w324:dbl, "X Scale"=w323:cluster{"Xo":dbl, "delta X":dbl}, "X Max"=w322:dbl)
            n131 = Build Array(w334, w335) -> (w328:cluster{"min Z value":dbl, u32}[])
            n132 = property on="Inlet mapping" class="IntGraph (strict)"("Ignore Array"=FALSE, "ZScale.MarkerVals[]"=w328, "XScale.Ofst&Mult"=w325, "XScale.Maximum"=w324, "YScale.Ofst&Mult"=w323, "YScale.Maximum"=w322, "XScale.Precision"=w327, "YScale.Precision"=w327) -> ()  [unwired: 2 in, 2 out]
          }
          frame #2 {
            n133 = for {
              N: 5 -> [_]
              tunnel: w342 -> [w350]
              tunnel: w341 -> [w349]
              tunnel: [w344] -> w339 mode=indexing
              i -> [w346]
              w348 = 7 ("length")
              n134 = Multiply(x=w346, y=w348) -> (x*y=w347:i32)
              n135 = Array Subset(array=w349, index=w347, length=w348) -> (w345:dbl[])
              n136 = Bundle("Y Axis Current"=w350, w345) -> (w344:cluster{"Y Axis Current":dbl[], dbl[]})  [unwired: 1 in]
            }
            n137 = local read "Loop number"() -> (w337:i32)
            n138 = Reverse 1D Array(array=w339) -> (reversed array=w338:cluster{"Y Axis Current":dbl[], dbl[]}[])
            n139 = case shown="1, Default" w337 {
              tunnel: w338 -> [_ w343]
              frame 0 {
              }
              frame 1, Default {
                "Lateral profiles" <- w343
              }
            }
          }
        }
        n140 = Build Array (concatenate)(w280, w277) -> (w281:string[])
      }
      frame "EnFlo_Tunnel:Chiller_Pump:Enable" {
        n141 = Array Size(array=w361) -> (size(s)=w359:i32)
        n142 = Index Array(array=w358, index=w359) -> (element=w356:dbl)
        n143 = Greater?(x=w356, y=0.5) -> (0:→"Chiller_Pump:Enable":bool)
        n144 = Build Array (concatenate)(w361, "EnFlo_Tunnel:Chiller_Pump:Enable" ("Ch Name")) -> (w362:string[])
      }
      frame "EnFlo_Tunnel Chilled Water info" {
        n145 = Array Size(array=w390) -> (size(s)=w384:i32)
        n146 = Array Subset(array=w385, index=w384) -> (w383:dbl[])  [unwired: 1 in]
        n147 = Index Array(array=w383) -> (element #1=→"Supply Temp":dbl, element #2=→"Return Temp":dbl, element #3=→"Dem Temp":dbl, element #4=→"Mixing Valve %":dbl, element #5=w371:dbl, element #6=w370:dbl, element #7=→"Heat Exchanger Valve %":dbl, element #8=→"Exit Dem Temp":dbl, element #9=w376:dbl, element #10=w375:dbl, element #11=w367:dbl, element #12=w366:dbl)  [unwired: 12 in]
        "Supply Pressure" <- w376
        "Return Pressure" <- w375
        n148 = Multiply(x=w367, y=10.0) -> (x*y=→"Pump Speed %":dbl)
        n149 = Greater?(x=w366, y=0.5) -> (0:→"Chiller_Pump Running":bool)
        n150 = Max & Min(x=w371, y=w370) -> (max(x,y)=→"Max Motor Temp":dbl)  [unwired: 1 out]
        n151 = Build Array (concatenate)(w390, string[] ["EnFlo_Tunnel:Chilled Water:Supply", "EnFlo_Tunnel:Chilled Water:Return", "EnFlo_Tunnel:Chilled Water:Dem Temp", "EnFlo_Tunnel:Chilled Water:Valve Dem Pos", "EnFlo_Tunnel:Chilled Water:Motor1 Temp", "EnFlo_Tunnel:Chilled Water:Motor2 Temp", "EnFlo_Tunnel:Heat_Ex_Div_Valve:Dem Pos", "EnFlo_Tunnel:Exit Duct:Dem Temp", "EnFlo_Tunnel:Chilled Water:Pressure_supply (Bar)", "EnFlo_Tunnel:Chilled Water:Pressure_return (Bar)", "EnFlo_Tunnel:Chilled Water:Motor_Dem_Voltage", "EnFlo_Tunnel:Chiller_Pump:Running"] ("subarray")) -> (w391:string[])
        n152 = Subtract(x=w376, y=w375) -> (x-y=→"Meas Delta P":dbl)
      }
      frame "EnFlo_Tunnel:Floor_Cooling:Enable" {
        n153 = Array Size(array=w403) -> (size(s)=w401:i32)
        n154 = Index Array(array=w400, index=w401) -> (element=w398:dbl)
        n155 = Greater?(x=w398, y=0.5) -> (0:→"Floor_Cooling:Enable":bool)
        n156 = Build Array (concatenate)(w403, "EnFlo_Tunnel:Floor_Cooling:Enable" ("Ch Name")) -> (w404:string[])
      }
      frame "Floor Panels Return Temps" {
        w420 = string[] ["EnFlo_Tunnel:Return_Temp:Floor_Far_02", "EnFlo_Tunnel:Return_Temp:Floor_Near_02", "EnFlo_Tunnel:Return_Temp:Floor_Far_03", "EnFlo_Tunnel:Return_Temp:Floor_Near_03", "EnFlo_Tunnel:Return_Temp:Floor_Far_04", "EnFlo_Tunnel:Return_Temp:Floor_Near_04", "EnFlo_Tunnel:Return_Temp:Floor_Far_05", "EnFlo_Tunnel:Return_Temp:Floor_Near_05", "EnFlo_Tunnel:Return_Temp:Floor_Far_06", "EnFlo_Tunnel:Return_Temp:Floor_Near_06", "EnFlo_Tunnel:Return_Temp:Floor_Far_07", "EnFlo_Tunnel:Return_Temp:Floor_Near_07", "EnFlo_Tunnel:Return_Temp:Floor_Far_08", "EnFlo_Tunnel:Return_Temp:Floor_Near_08", "EnFlo_Tunnel:Return_Temp:Floor_Far_09", "EnFlo_Tunnel:Return_Temp:Floor_Near_09", "EnFlo_Tunnel:Return_Temp:Floor_Far_10", "EnFlo_Tunnel:Return_Temp:Floor_Near_10", "EnFlo_Tunnel:Return_Temp:Floor_Far_11", "EnFlo_Tunnel:Return_Temp:Floor_Near_11", "EnFlo_Tunnel:Return_Temp:Floor_Far_12", "EnFlo_Tunnel:Return_Temp:Floor_Near_12", "EnFlo_Tunnel:Return_Temp:Floor_Far_13", "EnFlo_Tunnel:Return_Temp:Floor_Near_13", "EnFlo_Tunnel:Return_Temp:Floor_Far_14", "EnFlo_Tunnel:Return_Temp:Floor_Turn_14", "EnFlo_Tunnel:Return_Temp:Floor_Turn_Sur_14", "EnFlo_Tunnel:Return_Temp:Floor_Turn_Sur_15", "EnFlo_Tunnel:Return_Temp:Floor_Far_16", "EnFlo_Tunnel:Return_Temp:Floor_Near_16", "EnFlo_Tunnel:Return_Temp:Floor_Far_17", "EnFlo_Tunnel:Return_Temp:Floor_Near_17", "EnFlo_Tunnel:Return_Temp:Floor_Far_18", "EnFlo_Tunnel:Return_Temp:Floor_Near_18", "EnFlo_Tunnel:Return_Temp:Floor_Far_19", "EnFlo_Tunnel:Return_Temp:Floor_Near_19"] ("subarray")
        n157 = Array Size(array=w426) -> (size(s)=w425:i32)
        n158 = local read "Dem Temp"() -> (w414:dbl)
        n159 = for {
          N: 18 -> [_]
          tunnel: [w443] -> w415 mode=indexing
          tunnel: w414 -> [w441]
          tunnel: [w441] -> w413 mode=indexing
          i -> [w444]
          n160 = Add(x=1.5, y=w444) -> (x+y=w443:dbl)
        }
        n161 = Bundle(w415, w413) -> (w409:cluster{dbl[], dbl[]})  [unwired: 1 in]
        n162 = Array Size(array=w420) -> (size(s)=w424:i32)
        n163 = Array Subset(array=w423, index=w425, length=w424) -> (w419:dbl[])
        n164 = Decimate 1D Array(w419) -> (w410:dbl[], w418:dbl[])
        n165 = Not A Number/Path/Refnum?(number/path/refnum=w410) -> (NaN/Path/Refnum?=w412:bool[])
        n166 = And Array Elements(Boolean array=w412) -> (logical AND=w411:bool)
        n167 = Bundle(w415, w410) -> (w417:cluster{dbl[], dbl[]})  [unwired: 1 in]
        n168 = Bundle(w415, w418) -> (w416:cluster{dbl[], dbl[]})  [unwired: 1 in]
        n169 = Build Array(w417, w416, w409) -> (w407:cluster{dbl[], dbl[]}[])
        n170 = case shown="True" w411 {
          tunnel: w409 -> [_ w440]
          tunnel: [w435 w439] -> w408
          tunnel: w407 -> [w435 _]
          frame False {
            n171 = property on="Panel Temps" class="XYGraph (strict)"("Active Plot"=u32 0, "Plot.Plot Name"="Dem Water Temp", "Active Plot"=u32 1, "Plot.Plot Name"="Y-ve Floor Water Return", "Active Plot"=u32 2, "Plot.Plot Name"="Y+ve Floor Water Return") -> ()  [unwired: 2 in, 2 out]
          }
          frame True {
            n172 = property on="Panel Temps" class="XYGraph (strict)"("Active Plot"=u32 0, "Plot.Plot Name"="Dem Water Temp") -> ()  [unwired: 2 in, 2 out]
            n173 = Build Array(w440) -> (w439:cluster{dbl[], dbl[]}[])
          }
        }
        n174 = Build Array (concatenate)(w426, w420) -> (w427:string[])
      }
      frame "Roof Panel Values" {
        w448 = string[] ["EnFlo_Tunnel:Temp:Roof_Far_2", "EnFlo_Tunnel:Temp:Roof_Near_3", "EnFlo_Tunnel:Temp:Roof_Far_4", "EnFlo_Tunnel:Temp:Roof_Far_6", "EnFlo_Tunnel:Temp:Roof_Near_7", "EnFlo_Tunnel:Temp:Roof_Far_8", "EnFlo_Tunnel:Temp:Roof_Far_10", "EnFlo_Tunnel:Temp:Roof_Near_12", "EnFlo_Tunnel:Temp:Roof_Far_15", "EnFlo_Tunnel:Temp:Roof_Far_19"] ("subarray")
        n175 = Array Size(array=w456) -> (size(s)=w455:i32)
        n176 = Array Size(array=w448) -> (size(s)=w454:i32)
        n177 = Array Subset(array=w453, index=w455, length=w454) -> (w449:dbl[])
        n178 = Build Array (concatenate)(w456, w448) -> (w457:string[])
        n179 = Bundle(dbl[] [1.5, 2.5, 3.5, 5.5, 6.5, 7.5, 9.5, 11.5, 14.5, 18.5], w449) -> (w446:cluster{dbl[], dbl[]})  [unwired: 1 in]
        n180 = Build Array (concatenate)(w451, w446) -> (w450:cluster{dbl[], dbl[]}[])
      }
      frame "Floor Panel Temps" {
        w465 = string[] ["EnFlo_Tunnel:Temp:Floor_X=02m", "EnFlo_Tunnel:Temp:Floor_X=03m", "EnFlo_Tunnel:Temp:Floor_X=04m", "EnFlo_Tunnel:Temp:Floor_X=05m", "EnFlo_Tunnel:Temp:Floor_X=06m", "EnFlo_Tunnel:Temp:Floor_X=07m", "EnFlo_Tunnel:Temp:Floor_X=08m", "EnFlo_Tunnel:Temp:Floor_X=09m", "EnFlo_Tunnel:Temp:Floor_X=10m", "EnFlo_Tunnel:Temp:Floor_X=11m", "EnFlo_Tunnel:Temp:Floor_X=12m", "EnFlo_Tunnel:Temp:Floor_X=13m", "EnFlo_Tunnel:Temp:Floor_X=14m", "EnFlo_Tunnel:Temp:Floor_X=15m", "EnFlo_Tunnel:Temp:Floor_X=16m", "EnFlo_Tunnel:Temp:Floor_X=17m", "EnFlo_Tunnel:Temp:Floor_X=18m"] ("subarray")
        n181 = Array Size(array=w472) -> (size(s)=w471:i32)
        n182 = Array Size(array=w465) -> (size(s)=w470:i32)
        n183 = Array Subset(array=w469, index=w471, length=w470) -> (w467:dbl[])
        n184 = Build Array (concatenate)(w472, w465) -> (w473:string[])
        n185 = property on="Floor Panels" class="XYGraph (strict)"("Active Plot"=u32 0, "Plot.Plot Name"="Temp") -> ()  [unwired: 2 in, 2 out]
        n186 = Bundle("Array"=dbl[] [1.5, 2.5, 3.5, 4.5, 5.5, 6.5, 7.5, 8.5, 9.5, 10.5, 11.5, 12.5, 13.5, 14.5, 15.5, 16.5, 17.5], w467) -> (w463:cluster{"Array":dbl[], dbl[]})  [unwired: 1 in]
        n187 = Build Array(w463) -> (w462:cluster{"Array":dbl[], dbl[]}[])
      }
      frame "Floor Panel Setpoints" {
        w483 = string[] ["EnFlo_Tunnel:Setpoint:Floor_X=02m", "EnFlo_Tunnel:Setpoint:Floor_X=03m", "EnFlo_Tunnel:Setpoint:Floor_X=04m", "EnFlo_Tunnel:Setpoint:Floor_X=05m", "EnFlo_Tunnel:Setpoint:Floor_X=06m", "EnFlo_Tunnel:Setpoint:Floor_X=07m", "EnFlo_Tunnel:Setpoint:Floor_X=08m", "EnFlo_Tunnel:Setpoint:Floor_X=09m", "EnFlo_Tunnel:Setpoint:Floor_X=10m", "EnFlo_Tunnel:Setpoint:Floor_X=11m", "EnFlo_Tunnel:Setpoint:Floor_X=12m", "EnFlo_Tunnel:Setpoint:Floor_X=13m", "EnFlo_Tunnel:Setpoint:Floor_X=14m", "EnFlo_Tunnel:Setpoint:Floor_X=15m", "EnFlo_Tunnel:Setpoint:Floor_X=16m", "EnFlo_Tunnel:Setpoint:Floor_X=17m", "EnFlo_Tunnel:Setpoint:Floor_X=18m"] ("subarray")
        n188 = Array Size(array=w489) -> (size(s)=w488:i32)
        n189 = Array Size(array=w479) -> (size(s)=w478:i32)
        n190 = Array Size(array=w483) -> (size(s)=w487:i32)
        n191 = Array Subset(array=w486, index=w488, length=w487) -> (w484:dbl[])
        n192 = Build Array (concatenate)(w489, w483) -> (w490:string[])
        n193 = property on="Floor Panels" class="XYGraph (strict)"("Active Plot"=w478, "Plot.Plot Name"="Setpoint") -> ()  [unwired: 2 in, 2 out]
        n194 = Bundle("Array"=dbl[] [1.5, 2.5, 3.5, 4.5, 5.5, 6.5, 7.5, 8.5, 9.5, 10.5, 11.5, 12.5, 13.5, 14.5, 15.5, 16.5, 17.5], w484) -> (w481:cluster{"Array":dbl[], dbl[]})  [unwired: 1 in]
        n195 = Build Array (concatenate)(w479, w481) -> (w480:cluster{"Array":dbl[], dbl[]}[])
      }
      frame "Floor Panel Powers" {
        w500 = string[] ["EnFlo_Tunnel:Power:Floor_X=02m", "EnFlo_Tunnel:Power:Floor_X=03m", "EnFlo_Tunnel:Power:Floor_X=04m", "EnFlo_Tunnel:Power:Floor_X=05m", "EnFlo_Tunnel:Power:Floor_X=06m", "EnFlo_Tunnel:Power:Floor_X=07m", "EnFlo_Tunnel:Power:Floor_X=08m", "EnFlo_Tunnel:Power:Floor_X=09m", "EnFlo_Tunnel:Power:Floor_X=10m", "EnFlo_Tunnel:Power:Floor_X=11m", "EnFlo_Tunnel:Power:Floor_X=12m", "EnFlo_Tunnel:Power:Floor_X=13m", "EnFlo_Tunnel:Power:Floor_X=14m", "EnFlo_Tunnel:Power:Floor_X=15m", "EnFlo_Tunnel:Power:Floor_X=16m", "EnFlo_Tunnel:Power:Floor_X=17m", "EnFlo_Tunnel:Power:Floor_X=18m"] ("subarray")
        n196 = Array Size(array=w506) -> (size(s)=w505:i32)
        n197 = Array Size(array=w496) -> (size(s)=w495:i32)
        n198 = Array Size(array=w500) -> (size(s)=w504:i32)
        n199 = Array Subset(array=w503, index=w505, length=w504) -> (w501:dbl[])
        n200 = Build Array (concatenate)(w506, w500) -> (w507:string[])
        n201 = property on="Floor Panels" class="XYGraph (strict)"("Active Plot"=w495, "Plot.Plot Name"="Power") -> ()  [unwired: 2 in, 2 out]
        n202 = Bundle("Array"=dbl[] [1.5, 2.5, 3.5, 4.5, 5.5, 6.5, 7.5, 8.5, 9.5, 10.5, 11.5, 12.5, 13.5, 14.5, 15.5, 16.5, 17.5], w501) -> (w498:cluster{"Array":dbl[], dbl[]})  [unwired: 1 in]
        n203 = Build Array (concatenate)(w496, w498) -> (w497:cluster{"Array":dbl[], dbl[]}[])
      }
      frame "Lab Stratification" {
        w527 = dbl[] [0.0, 6.0]
        w530 = 8 ("length")
        w542 = dbl[] [5.75, 4.5, 3.5, 2.5, 1.5, 0.5, 0.1, 0.0]
        n204 = Array Size(array=w545) -> (size(s)=w529:i32)
        n205 = Add(x=w529, y=w530) -> (x+y=w528:i32)
        n206 = Array Subset(array=w532, index=w528) -> (w531:dbl[])  [unwired: 1 in]
        n207 = Index Array(array=w531) -> (element #1=→"Delta T":dbl, element #2=w524:dbl, element #3=→"Heat Extraction kW":dbl, element #4=w526:dbl, element #5=→"Inlet_Temp Average":dbl)  [unwired: 5 in]
        "Lab Reference Temp" <- w524
        "Des Air Temp" <- w526
        n208 = Array Subset(array=w532, index=w529, length=w530) -> (w535:dbl[])
        n209 = for {
          N: 15 -> [_]
          tunnel: 2.43 -> [w553]
          tunnel: [w551] -> w539 mode=indexing
          i -> [w555]
          n210 = Multiply(x=0.1, y=w555) -> (x*y=w552:dbl)
          n211 = Subtract(x=w553, y=w552) -> (x-y=w551:dbl)
        }
        n212 = call <vilib>:"Interpolate 1D.vi"("xi"=w539, "X"=w542, "Y"=w535) -> ("yi"=w538:dbl[])  [unwired: 3 in, 5 out]
        n213 = Build Array(w526, w526) -> (w525:dbl[])
        n214 = Build Array(w524, w524) -> (w523:dbl[])
        n215 = local read "Heaters Enabled"() -> (w514:bool)
        n216 = Bundle(w535, w542) -> (w522:cluster{dbl[], dbl[]})  [unwired: 1 in]
        n217 = Bundle(w525, w527) -> (w521:cluster{dbl[], dbl[]})  [unwired: 1 in]
        n218 = Bundle(w523, w527) -> (w520:cluster{dbl[], dbl[]})  [unwired: 1 in]
        n219 = Bundle("yi"=w538, w518) -> (w537:cluster{"yi":dbl[], dbl[]})  [unwired: 1 in]
        n220 = case shown="False" w514 {
          tunnel: ["Get Server Values" "Inlet Heater Setpoint Values"] -> w513
          frame False {
          }
          frame True {
          }
        }
        n221 = Build Array(w522, w521, w520) -> (w519:cluster{dbl[], dbl[]}[])
        n222 = Build Array (concatenate)(w545, string[] ["EnFlo Lab:labstrat1:Z=5.75m Roof", "EnFlo Lab:labstrat1:Z=4.5m", "EnFlo Lab:labstrat1:Z=3.5m", "EnFlo Lab:labstrat1:Z=2.5m", "EnFlo Lab:labstrat1:Z=1.5m", "EnFlo Lab:labstrat1:Z=0.5m", "EnFlo Lab:labstrat1:Z=0.1m", "EnFlo Lab:labstrat1:Z=0m Floor", "EnFlo Lab:labstrat1:Delta T", "EnFlo_Lab:Reference:Temperature", "EnFlo Lab:Heat:Extraction", "EnFlo Lab:Desired:Air Temp", "EnFlo_Tunnel:Inlet_Temp:Average"] ("subarray")) -> (w546:string[])
        n223 = local read "Loop number"() -> (w512:i32)
        n224 = case shown="1, Default" w512 {
          tunnel: w519 -> [_ w548]
          frame 0 {
          }
          frame 1, Default {
            "Strat" <- w548
          }
        }
        n225 = Array Size(array=w515) -> (size(s)=w516:i32)
        n226 = Build Array (concatenate)(w515, w537) -> (w536:cluster{"yi":dbl[], dbl[]}[])
        n227 = property on="Inlet Heaters" class="XYGraph (strict)"("Active Plot"=w516, "Plot.Plot Name"="Lab Strat") -> ()  [unwired: 2 in, 2 out]
      }
      frame "Inlet Heater Setpoint Values" {
        w557 = string[] ["EnFlo_Tunnel:Setpoint:Inlet_Y=0_Z=1450", "EnFlo_Tunnel:Setpoint:Inlet_Y=0_Z=1350", "EnFlo_Tunnel:Setpoint:Inlet_Y=0_Z=1250", "EnFlo_Tunnel:Setpoint:Inlet_Y=0_Z=1150", "EnFlo_Tunnel:Setpoint:Inlet_Y=0_Z=1050", "EnFlo_Tunnel:Setpoint:Inlet_Y=0_Z=950", "EnFlo_Tunnel:Setpoint:Inlet_Y=0_Z=850", "EnFlo_Tunnel:Setpoint:Inlet_Y=0_Z=750", "EnFlo_Tunnel:Setpoint:Inlet_Y=0_Z=650", "EnFlo_Tunnel:Setpoint:Inlet_Y=0_Z=550", "EnFlo_Tunnel:Setpoint:Inlet_Y=0_Z=450", "EnFlo_Tunnel:Setpoint:Inlet_Y=0_Z=350", "EnFlo_Tunnel:Setpoint:Inlet_Y=0_Z=250", "EnFlo_Tunnel:Setpoint:Inlet_Y=0_Z=150", "EnFlo_Tunnel:Setpoint:Inlet_Y=0_Z=50"] ("subarray")
        n228 = Array Size(array=w572) -> (size(s)=w571:i32)
        n229 = Array Size(array=w560) -> (size(s)=w558:i32)
        n230 = property on="Inlet Heaters" class="XYGraph (strict)"("Active Plot"=w558, "Plot.Plot Name"="Inlet Setpoints") -> ()  [unwired: 2 in, 2 out]
        n231 = Array Size(array=w557) -> (size(s)=w570:i32)
        n232 = Array Subset(array=w569, index=w571, length=w570) -> (w562:dbl[])
        n233 = Bundle(w562, w561) -> (w568:cluster{dbl[], dbl[]})  [unwired: 1 in]
        n234 = for {
          tunnel: i32[] [14, 10, 5, 0] -> [w577] mode=indexing
          tunnel: w562 -> [w575]
          tunnel: [w576] -> w564 mode=indexing
          n235 = Index Array(array=w575, index=w577) -> (element=w576:dbl)
        }
        "Setpoints" <- w564
        n236 = Build Array (concatenate)(w572, w557) -> (w573:string[])
        n237 = Build Array (concatenate)(w560, w568) -> (w567:cluster{"yi":dbl[], dbl[]}[])
      }
      frame "Inlet Heater Power Values" {
        w579 = string[] ["EnFlo_Tunnel:Power:Inlet_Y=0_Z=1450", "EnFlo_Tunnel:Power:Inlet_Y=0_Z=1350", "EnFlo_Tunnel:Power:Inlet_Y=0_Z=1250", "EnFlo_Tunnel:Power:Inlet_Y=0_Z=1150", "EnFlo_Tunnel:Power:Inlet_Y=0_Z=1050", "EnFlo_Tunnel:Power:Inlet_Y=0_Z=950", "EnFlo_Tunnel:Power:Inlet_Y=0_Z=850", "EnFlo_Tunnel:Power:Inlet_Y=0_Z=750", "EnFlo_Tunnel:Power:Inlet_Y=0_Z=650", "EnFlo_Tunnel:Power:Inlet_Y=0_Z=550", "EnFlo_Tunnel:Power:Inlet_Y=0_Z=450", "EnFlo_Tunnel:Power:Inlet_Y=0_Z=350", "EnFlo_Tunnel:Power:Inlet_Y=0_Z=250", "EnFlo_Tunnel:Power:Inlet_Y=0_Z=150", "EnFlo_Tunnel:Power:Inlet_Y=0_Z=50"] ("subarray")
        n238 = Array Size(array=w592) -> (size(s)=w591:i32)
        n239 = Array Size(array=w581) -> (size(s)=w582:i32)
        n240 = Array Size(array=w579) -> (size(s)=w590:i32)
        n241 = Array Subset(array=w589, index=w591, length=w590) -> (w588:dbl[])
        n242 = Bundle(w588, w586) -> (w584:cluster{dbl[], dbl[]})  [unwired: 1 in]
        n243 = Build Array (concatenate)(w592, w579) -> (w593:string[])
        n244 = property on="Inlet Heaters" class="XYGraph (strict)"("Active Plot"=w582, "Plot.Plot Name"="Inlet Powers") -> ()  [unwired: 2 in, 2 out]
        n245 = Build Array (concatenate)(w581, w584) -> (w585:cluster{"yi":dbl[], dbl[]}[])
      }
      frame "Get Server Values" {
        n246 = local read "Loop number"() -> (w600:i32)
        n247 = Increment(x=w600) -> (x+1=w604:i32)
        n248 = local write "Loop number"(w604) -> ()
        n249 = case shown="1" w600 {
          tunnel: w603 -> [_ w621 _]
          tunnel: [TRUE ("Top Level") w619 w640] -> w606
          frame 0 {
          }
          frame 1 {
            n250 = for {
              tunnel: T2 {"Template Channel Name"="", "Description"="", "Tolerance"=0.0, "Precision"="", "Folder level"="", "Source"=[], "Replace"=[], "Summarise"=FALSE, "Min Value"="", "Maths"="", "Omit Rows Containing"=[], "Ignore When"=[], "Max Value"="", "Dispose"=enum."Always"} ("Cluster") -> [w630]
              tunnel: w621 -> [w623] mode=indexing
              tunnel: [w629] -> w617 mode=indexing if=w625
              shift-right: [w627] -> _
              shift-left: string[] [] -> [w628]
              tunnel: "Do not prompt me if this channnel is not found" -> [w622]
              n251 = Search 1D Array(1D array=w628, element=w623) -> (index of element=w626:i32)  [unwired: 1 in]
              n252 = Build Array(w623, w622) -> (w624:string[])
              n253 = Bundle By Name(cluster=w630, "Template Channel Name"=w623, "Source"=w624) -> (w629:T2)
              n254 = case shown="Default" w626 {
                tunnel: w628 -> [w632 w636]
                tunnel: [w632 w635] -> w627
                tunnel: w623 -> [_ w634]
                tunnel: [FALSE TRUE] -> w625
                frame Default {
                }
                frame -1 {
                  n255 = Build Array (concatenate)(w636, w634) -> (w635:string[])
                }
              }
            }
            n256 = global read "Constants_global.vi" "Data Folder Local"() -> (w620:path)
            n257 = Build Path(base path=w620, name or relative path="EnFlo_Tunnel_Display_Template.xls") -> (appended path=w613:path)
            n258 = local read "Top Level"() -> (w619:bool)
            n259 = call "Read_Write_Temp_Cluster.vi"("Template Info Array"=w617, "Mode"=Global_mode."Write Global to File", "Template File"=w613) -> ()  [unwired: 2 in, 1 out]
          }
          frame Default {
            n260 = global read "Results_plotter_Global.vi" "Plot EnFlo Tunnel Display"() -> (w639:bool)
            n261 = Or(x=w639, y="Stop Button") -> (x .or. y?=w637:bool)
            n262 = Not(x=w637) -> (.not. x?=w640:bool)
          }
        }
        n263 = Multiply(x="History in Minutes", y=60.0) -> (x*y=w597:dbl)
        n264 = call "Get_Channel_averages.vi"("Desired Ch Names"=w603, "Averaging time (mins)"="Averaging time (mins)", "End Offset Sec (0)"=w597) -> ("number"=w605:dbl[])  [unwired: 2 out]
        n265 = case shown="1, Default" w600 {
          tunnel: w602 -> [_ w610]
          tunnel: w601 -> [_ w609]
          tunnel: w599 -> [_ w608]
          frame 0 {
          }
          frame 1, Default {
            "Inlet Heaters" <- w609
            "Panel Temps" <- w610
            "Floor Panels" <- w608
          }
        }
      }
    }
  }
